vi "RT_VS50_Dynamics_DLR_v10_v11_PXI.vi"() -> ()   [LabVIEW 2017]
uses:
  <vilib>/Platform/TimedLoop/XDataNode/timing_clust.ctl
  <vilib>/Platform/TimedLoop/XDataNode/nitl_modes.ctl
  <vilib>/Platform/TimedLoop/XDataNode/wakeup.ctl
  <vilib>/Analysis/coordinate.llb/Euler Rotation Order.ctl
  <vilib>/Analysis/_algsub.llb/Vector Norm Type.ctl
  <vilib>/DAQmx/read.llb/DAQmx Read (Analog DBL 1Chan 1Samp).vi
  <vilib>/DAQmx/write.llb/DAQmx Write (Analog DBL 1Chan 1Samp).vi
  <vilib>/Analysis/baseanly.llb/Real A x B.vi
  <vilib>/Analysis/_algsub.llb/Real Vector Norm.vi
  <vilib>/Instr/_visa.llb/VISA Configure Serial Port (Instr).vi
  <vilib>/Utility/file.llb/Read Delimited Spreadsheet (DBL).vi
  <vilib>/DAQmx/create/channels.llb/DAQmx Create Channel (AO-Voltage-Basic).vi
  <vilib>/DAQmx/create/channels.llb/DAQmx Create Channel (AI-Voltage-Basic).vi
  <vilib>/DAQmx/miscellaneous.llb/DAQmx Fill In Error Info.vi
  <vilib>/Analysis/Matrix/Numeric/Conversions/Array To Matrix - RA2.vi
  <vilib>/Analysis/Matrix/Numeric/Conversions/Array To Matrix - RA.vi
  <vilib>/Analysis/Matrix/Numeric/Conversions/Matrix To Array - RM.vi
  <vilib>/Platform/TimedLoop/XDataNode/XDataNode.xnode
  <vilib>/Analysis/NI_AALPro.lvlib
  <vilib>/Platform/TimedLoop/XDataNode/XDNodeRunTimeDep.lvlib
  <vilib>/Utility/file.llb/Read From Spreadsheet File (DBL).vi
  <vilib>/Analysis/Matrix/NI_Matrix.lvlib
  <vilib>/Analysis/NI_AALBase.lvlib
  <vilib>/ptbypt/NI_PtbyPt.lvlib
panel:
  out "e (i+1)":cluster{dbl[], dbl[]}[](graph)
  out "all rows 2":dbl[][](array[numeric]) format="%0.3f"
  out "PID_array":dbl[][](array[numeric])
  in  "Guiamento":bool
  in  "Debug":bool
  in  "BR ACT - oscillation pitch":bool
  in  "BR ACT - oscillation yaw":bool
  in  "Amplitude [deg]":dbl=4.0 format="%#_13g"
  in  "Frequency [Hz]":dbl=1.0 format="%#_13g"
  out "BR ACT enable":bool
  in  "BR ACT - Enable Manual cmd":bool
  out "ACT Pitch [deg] mean":dbl format="%0.2f"
  out "ACT Yaw [deg] mean":dbl format="%0.2f"
  out "ACT Pitch [deg]":dbl
  out "ACT Yaw [deg]":dbl
  out "mean y":dbl format="%0.2f"
  out "mean x":dbl format="%0.2f"
  out "Incl angle Y [deg]":dbl
  out "Incl angle X [deg]":dbl
  out "Iteration Duration LOG":i64
  out "Iteration Duration CFG CFN":i64
  out "Iteration Duration NAV CFN":i64
  out "Iteration Duration sim [us]":i64
  out "LOG Enable":bool
  out "Table enable":bool
  out "DMARS Enable":bool
  out "TVA Enable":bool
  out "CFN-61G Enable":bool
  out "CRC?":bool
  out "string out":string
  in  "STIM300 Enable":bool
  out "CRC OK":bool
  out "IMU accel status":u8 format="%b"
  out "IMU incl status":u8 format="%b"
  out "Samples Counter":u8
  out "IMU gyro status":u8 format="%b"
  out "Inc X [g]":dbl
  out "Inc Y [g]":dbl
  out "Inc Z [g]":dbl
  out "Iteration Duration STIM":i64
  out "ACT Pitch read":dbl(slide) scale=0.0..5.0
  out "ACT Yaw read":dbl(slide) scale=0.0..5.0
  in  "Atuador Yaw [Deg]":dbl(knob) scale=-4.0..4.0
  in  "Atuador Pitch [Deg]":dbl(knob) scale=-4.0..4.0
  out "Iteration Duration ACT":i64
  in  "Simulation Parameters":T1={"Wind VelocityAzimuth [deg] "=0.0, "Wind Velocity Module [m/s]"=0.0, "Fe gain"=1.0, "Cnalpha gain"=1.0, "clp gain"=1.0, "cld gain"=1.0, "cmq gain"=1.0, "cnr gain"=1.0, "dl [º]"=0.0, "Nozzle misalignment yaw/pitch [º]"=[0.0, 0.0], "Nozzle eccentricity x/y [m]"=[], "Wind_Profile"=0} {"Wind_Profile" min=0 max=3 step=1; "Wind Velocity Module [m/s]" format="%#_13g"; "Wind VelocityAzimuth [deg]" format="%#_13g"}
  in  "Initialization Parameters":T2={"W_b ini [rad/s]"=[0.0, 0.0, 0.0], "W ini [rad/s]"=[0.0, 0.0, 0.0], "altitude_ini(m)"=50.0, "lon_ini [º]"=-44.36778, "latd_ini [º]"=-2.31599, "V_ini [m/s]"=[0.0, 0.0, 0.0], "Initial Euler Angles [deg]"=[0.0, 0.0, 0.0], "CFN-61G Enable"=FALSE, "Table enable"=FALSE, "DMARS Enable"=FALSE, "German TVA Enable"=FALSE, "Sim_Time [s]"=82.0, "Control Selection"=enum."Sim Control", "LOG Enable"=FALSE, "BR ACT enable"=FALSE}
  out "concatenated string 2":string
  out "PXI log path 2":path
  out "concatenated string":string
  out "appended path":path
  in  "UTC format":bool
  out "spreadsheet string":string
  out "Sim_Time [s]":dbl
  in  "Rotation":T3
  out "TVA_cmd [deg] 2":dbl[](array[numeric])
  out "Control Variables (extra variables)":dbl[](array[numeric])
  in  "Send":bool
  out "Table Ready":bool
  out "CIVITA as DMARS [º]":cluster{"phi":dbl, "theta":dbl, "psi":dbl}
  in  "Cluster":T4={"Offset Roll"=0.0, "Offset Pitch"=0.0, "Offset Heading"=0.0, "Azimuth"=0.0, "Latitude "=-23.213156, "Longitude"=-45.860622, "Height"=622.367, "LP_Vel_Z-North"=0.0, "LP_Vel_Y-East"=0.0, "LP_Vel_X-Up"=0.0}
  out "Table cmd [º] inner middle outer":dbl[](array[numeric])
  out "DMARS SIM pred[º]":cluster{"phi":dbl, "theta":dbl, "psi":dbl}
  out "Control Variables\n (extra variables)":dbl[](array[numeric])
  out "ACT 315 Angle \"Yaw\"":dbl(slide) scale=-3.0..3.0
  out "ACT 225 Angle \"Pitch\"":dbl(slide) scale=-3.0..3.0
  out "TVA string 2":string
  out "TVA bytes read 2":u32
  out "CRC Check over Byte #10 to byte #84":bool
  out "CRC Check over Byte #2 to Byte #7 TVA2BComp":bool
  out "Iteration Duration TBL":i64
  out "Roll Rate/angle":dbl[](array[numeric])
  out "CRC Check over Byte #2 to Byte #7":bool
  out "CRC Check over Byte #10 to byte #29":bool
  out "GC_Counter 2":u32
  out "string to write DMARS":string="*IDN?"
  out "TVA string":string
  out "TVA bytes read":u32
  out "TVA sync bytes":string
  out "Time (s)":dbl
  out "POS":cluster{dbl, dbl, dbl} {"?" format="%_6g"; "?" format="%#1_6g"}
  out "RATE":cluster{dbl, dbl, dbl} {"?" format="%1_6g"}
  out "ACCEL":cluster{dbl, dbl, dbl} {"?" format="%1_6g"}
  out "Period":i64
  out "string enviada para acutrol":string
  in  "Remote Host":string="192.168.53.1"
  out "XYZ - rate_CIVITA":sgl[](array[numeric])
  out "Opp_Mode_CIVITA":string
  in  "NavOn":bool
  in  "Init":bool
  out "Long_Lat_Alt_CIVITA":sgl[](array[numeric])
  out "Euler Angles_CIVITA":sgl[](array[numeric])
  out "all rows":dbl[][](array[numeric]) format="%0.3f"
  in  "Start_SIMULATION":bool
  out "Data 4":dbl[][](array[numeric])
  out "Data 3":dbl[][](array[numeric])
  out "Data 2":dbl[][](array[numeric])
  out "Current time [s]":dbl
  out "bad iteration":bool
  in  "stop RT":bool
  out "SIM_Running":bool
  # "atitudes após leveling"
  # "0.279817"
  # "0.119821"
  # "0.24729"
  # "-0.038932"
  # "-0.0385253"
  # "-0.038247"
  # "-0.0193609"
  # "-0.0178696"
  # "-0.0176574"
  # "Posicão inicial"
  # "Posicao after 10min"
  # "-45.8606"
  # "-48.1427"
  # "-23.2132"
  # "-23.2324"
  # "0.622374"
  # "-4.67869"
  # "INS Civitanavi Control"
  # "0xAA/ 0x55"
  # "830 steps"
  # "Reiniciar a vi sempre antes de uma nova simulação!!"
  # "Simulation"
  # "TVA COMMUNICATIONS (German HW)"
  # "Enable buttons"
  # "Motion simulation table Control and Log files"
  # "Housekeeping data"
  # "º"
  # "Command Data"
  # "º"
  # "Km"
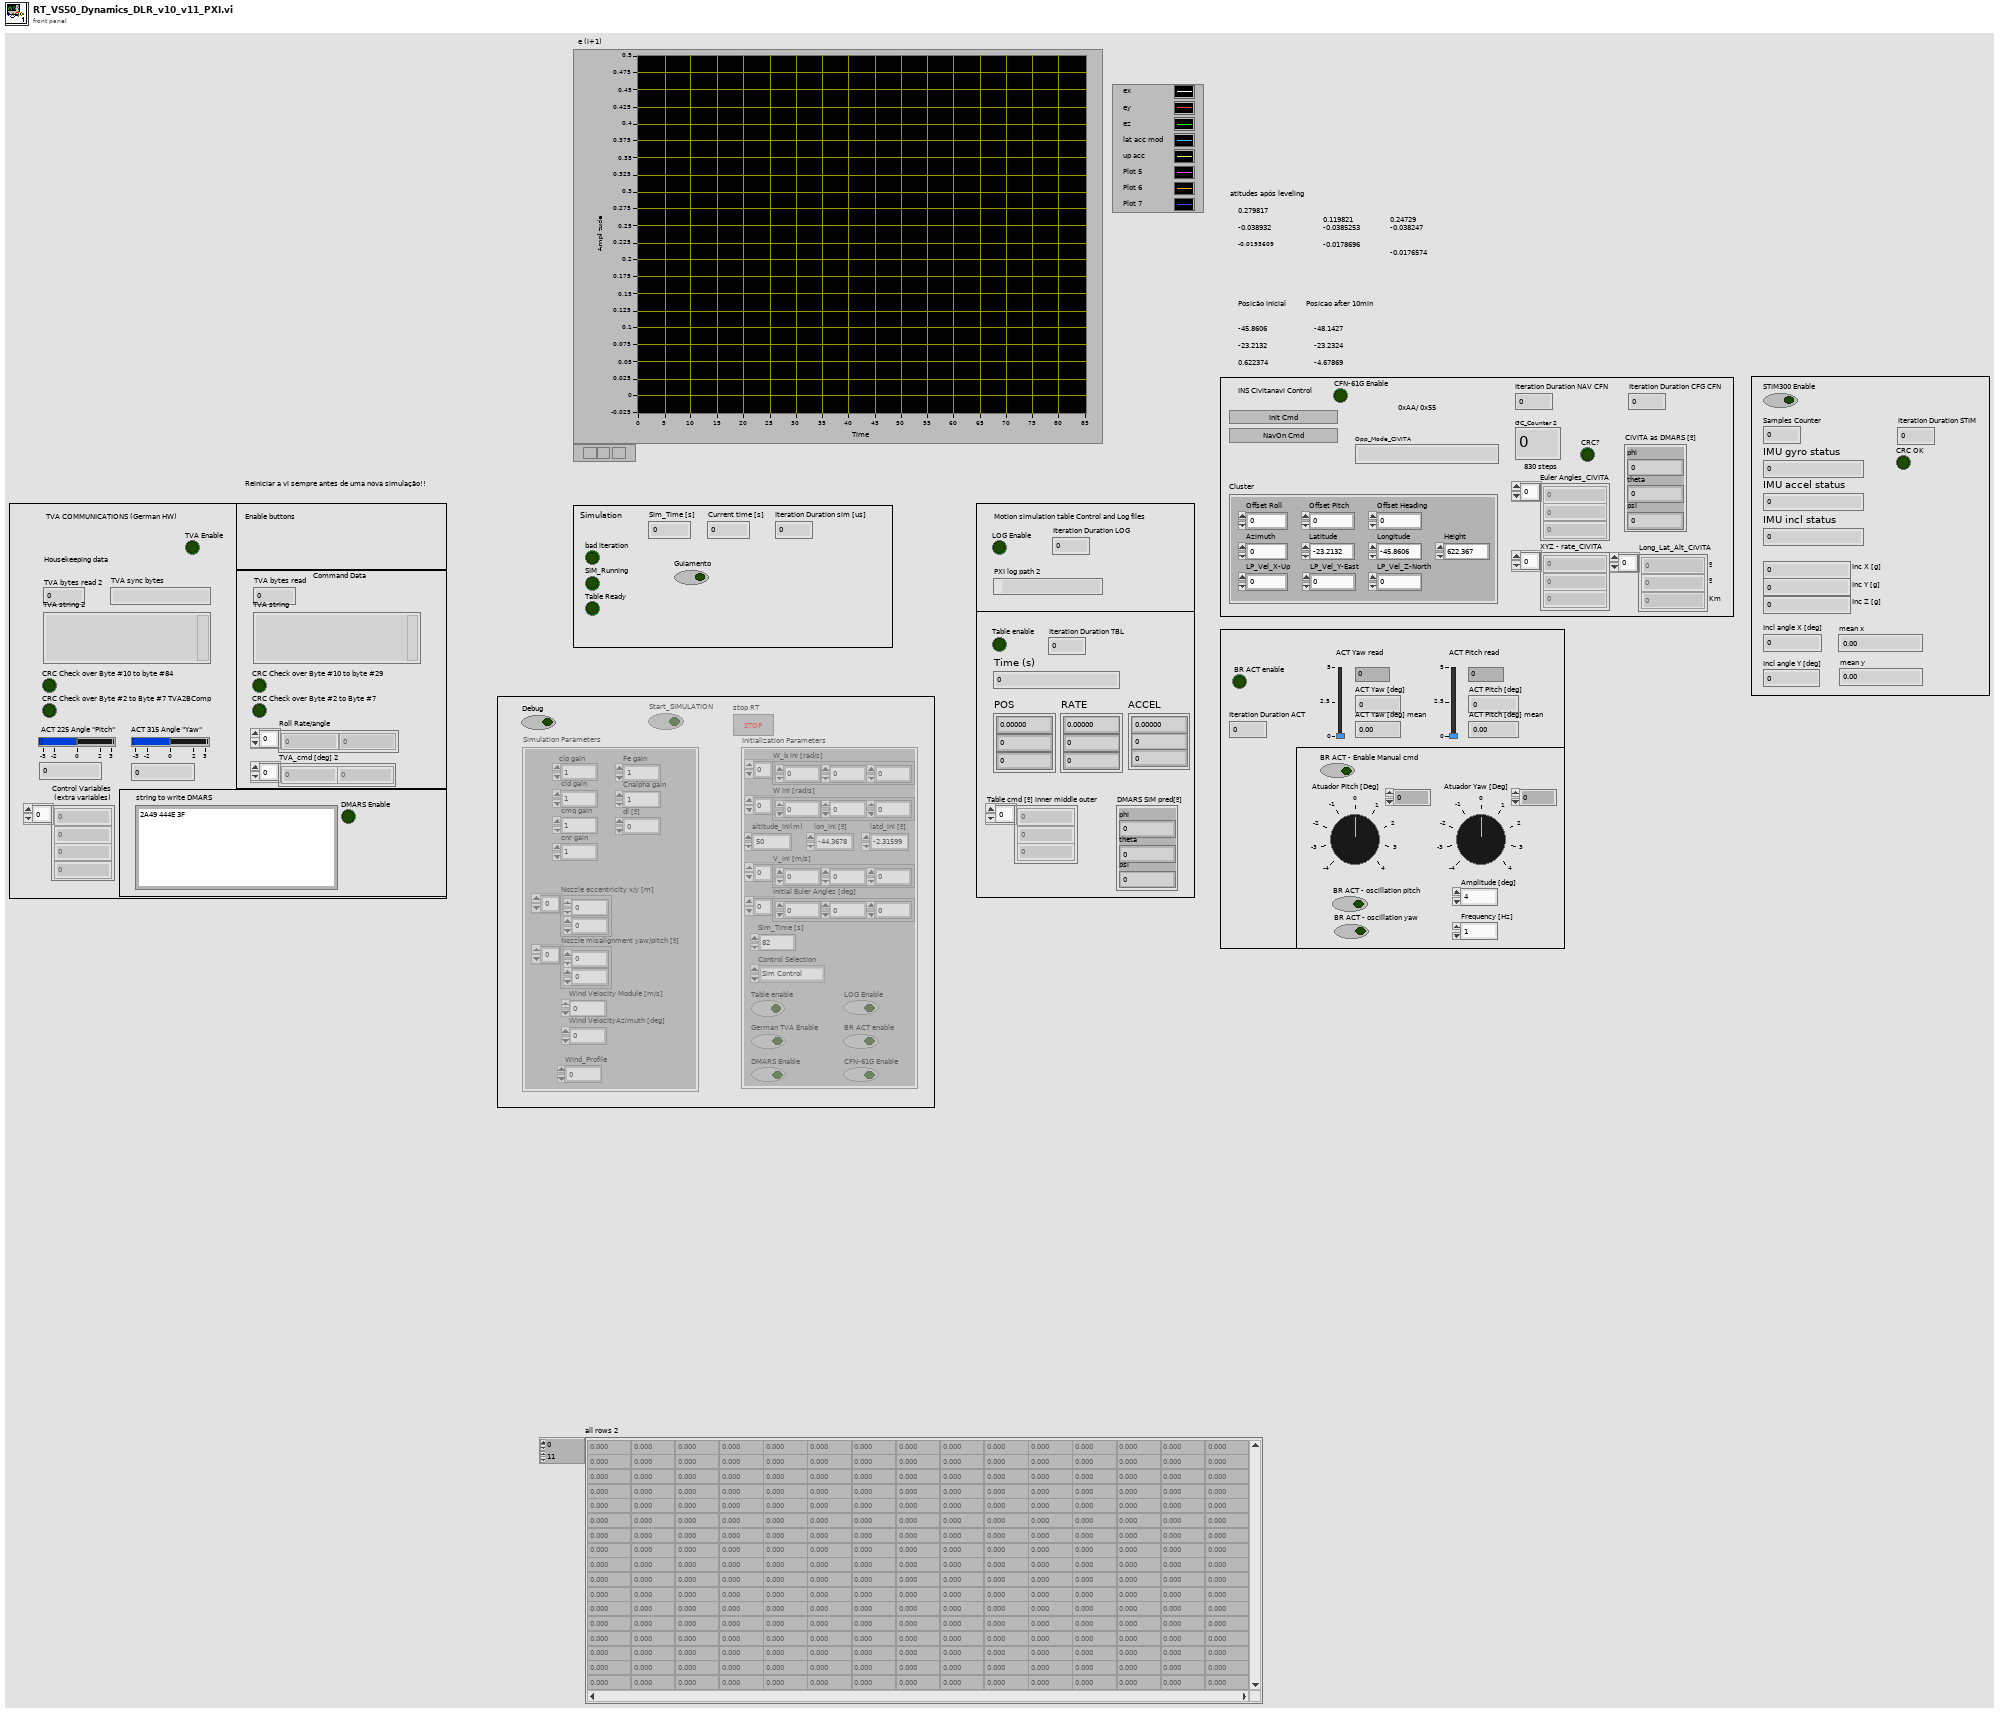
[diagram p1: front panel]
types:
  T1 = cluster{"Wind VelocityAzimuth [deg] ":dbl, "Wind Velocity Module [m/s]":dbl, "Fe gain":dbl, "Cnalpha gain":dbl, "clp gain":dbl, "cld gain":dbl, "cmq gain":dbl, "cnr gain":dbl, "dl [º]":dbl, "Nozzle misalignment yaw/pitch [º]":dbl[], "Nozzle eccentricity x/y [m]":dbl[], "Wind_Profile":i32}
  T2 = cluster{"W_b ini [rad/s]":dbl[], "W ini [rad/s]":dbl[], "altitude_ini(m)":dbl, "lon_ini [º]":dbl, "latd_ini [º]":dbl, "V_ini [m/s]":dbl[], "Initial Euler Angles [deg]":dbl[], "CFN-61G Enable":bool, "Table enable":bool, "DMARS Enable":bool, "German TVA Enable":bool, "Sim_Time [s]":dbl, "Control Selection":enum16{"Constant", "TVA E-BOX", "Sim Control"}, "LOG Enable":bool, "BR ACT enable":bool}
  T3 = cluster{"W(i) [rad/s]":dbl[], "W_b(i) [rad/s]":dbl[], "q(i)":dbl[], "Euler Angles {rad]":dbl[]}
  T4 = cluster{"Offset Roll":sgl, "Offset Pitch":sgl, "Offset Heading":sgl, "Azimuth":sgl, "Latitude ":sgl, "Longitude":sgl, "Height":sgl, "LP_Vel_Z-North":sgl, "LP_Vel_Y-East":sgl, "LP_Vel_X-Up":sgl}
  T5 = enum8{"Enabled", "Disabled", "Disabled and Grayed Out"}
  T6 = typedef "XDNodeRunTimeDep.lvlib/timing_clust.ctl" = cluster{"Expected End [f-1]":u64, "Actual End [f-1]":u64, "Finished Late? [f-1]":bool, "Expected End [i-1]":u64, "Actual End [i-1]":u64, "Finished Late? [i-1]":bool, "Expected Start [i]":u64, "Actual Start [i]":u64, "Expected Start [f]":u64, "Actual Start [f]":u64, "Source Name":string, "Structure Name":string, "Period":i64, "Deadline":i64, "Offset":i64, "Start":i64, "Priority":i32, "Timeout":i32, "Mode":T7, "Wakeup Reason":T8, "Error":errorcluster, "Source Type":string, "Secondary Source Type":string, "Global End Time":u64, "Global Start Time":u64, "Frame Duration":u64, "Iteration Duration":u64, "Assigned CPU":i32, "I/O Scan Engine Mode":u32}
  T7 = typedef "XDNodeRunTimeDep.lvlib/nitl_modes.ctl" = enum32{"No Change", "Process missed periods, maintain original phase", "Discard missed periods, maintain original phase", "Process missed periods, ignore original phase", "Discard missed periods, ignore original phase"}
  T8 = typedef "XDNodeRunTimeDep.lvlib/wakeup.ctl" = enum32{"Normal", "Aborted", "Asynchronous wakeup", "Timing source error", "Timed loop error", "Timeout"}
  T9 = cluster{"act_b [rad]":dbl[], "Oil Consumption [L]":dbl, "Act_b_TVA (315,225) [deg]":dbl[], "TVA cmd [rad]":dbl[], "BR ACT [rad]":dbl[]}
  T10 = cluster{"W(i+1) [rad/s]":dbl[], "W_b(i+1) [rad/s]":dbl[], "q(i+1)":dbl[], "Euler angles (i+1) XYZ [rad]":dbl[]}
  T11 = cluster{"position ECEF (i)":dbl[], "Lat_C [rad]":dbl, "latd(i+1) [rad]":dbl, "lon(i+1) [rad]":dbl, "height (i+1) [m]":dbl, "V(i+1) [m/s] NWU":dbl[]}
  T12 = cluster{"latd(i) [rad]":dbl, "lon(i) [rad]":dbl, "height(i)(m)":dbl, "V(i) [m/s] NWU":dbl[]}
  T13 = typedef "NI_AALPro.lvlib/Euler Rotation Order.ctl" = u16
  T14 = cluster{"dt [s]":dbl, "sim_running":bool, "t[s]":dbl, "i":i32}
  T15 = cluster{"Nzl_S [m^2]":dbl, "le [m]":dbl, "dl [rad]":dbl, "Dref[m]":dbl, "Sref [m^2]":dbl, "Nozzle misalignment yaw/pitch [º]":dbl[], "Nozzle eccentricity x/y [m]":dbl[]}
  T16 = typedef "NI_Matrix.lvlib/RealMatrix.ctl" = dbl[][]
  T17 = cluster{"output cluster":cluster{"AoA_pitch [rad]":dbl, "AoA_yaw [rad]":dbl, "Stream_direction [rad]":dbl[], "Speed_direction [rad]":dbl[]}, "M_alpha [rad/s^2], M_beta [rad/s^2]":cluster{"M_alpha [rad/s²]":dbl, "M_beta [rad/s²]":dbl}, "acc [m/s^2]":dbl[], "ang_acc":dbl[], "FE_b [N], FG [N], FA [N], Fco[N]":cluster{"FE_b [N]":dbl[], "FG [N]":dbl[], "FA [N]":dbl[], "Fco [N]":dbl[]}, "k_acc":cluster{"lat_acc_mod":dbl, "up_acc":dbl}}
  T18 = typedef "NI_AALPro.lvlib/Vector Norm Type.ctl" = u16
  T19 = enum16{"open", "replace", "create", "open or create", "replace or create", "replace or create with confirmation"}
  T20 = cluster{"Numeric":dbl, "upper limit":dbl, "upper limit":dbl}
  T21 = cluster{dbl, "upper limit":dbl, "upper limit":dbl}
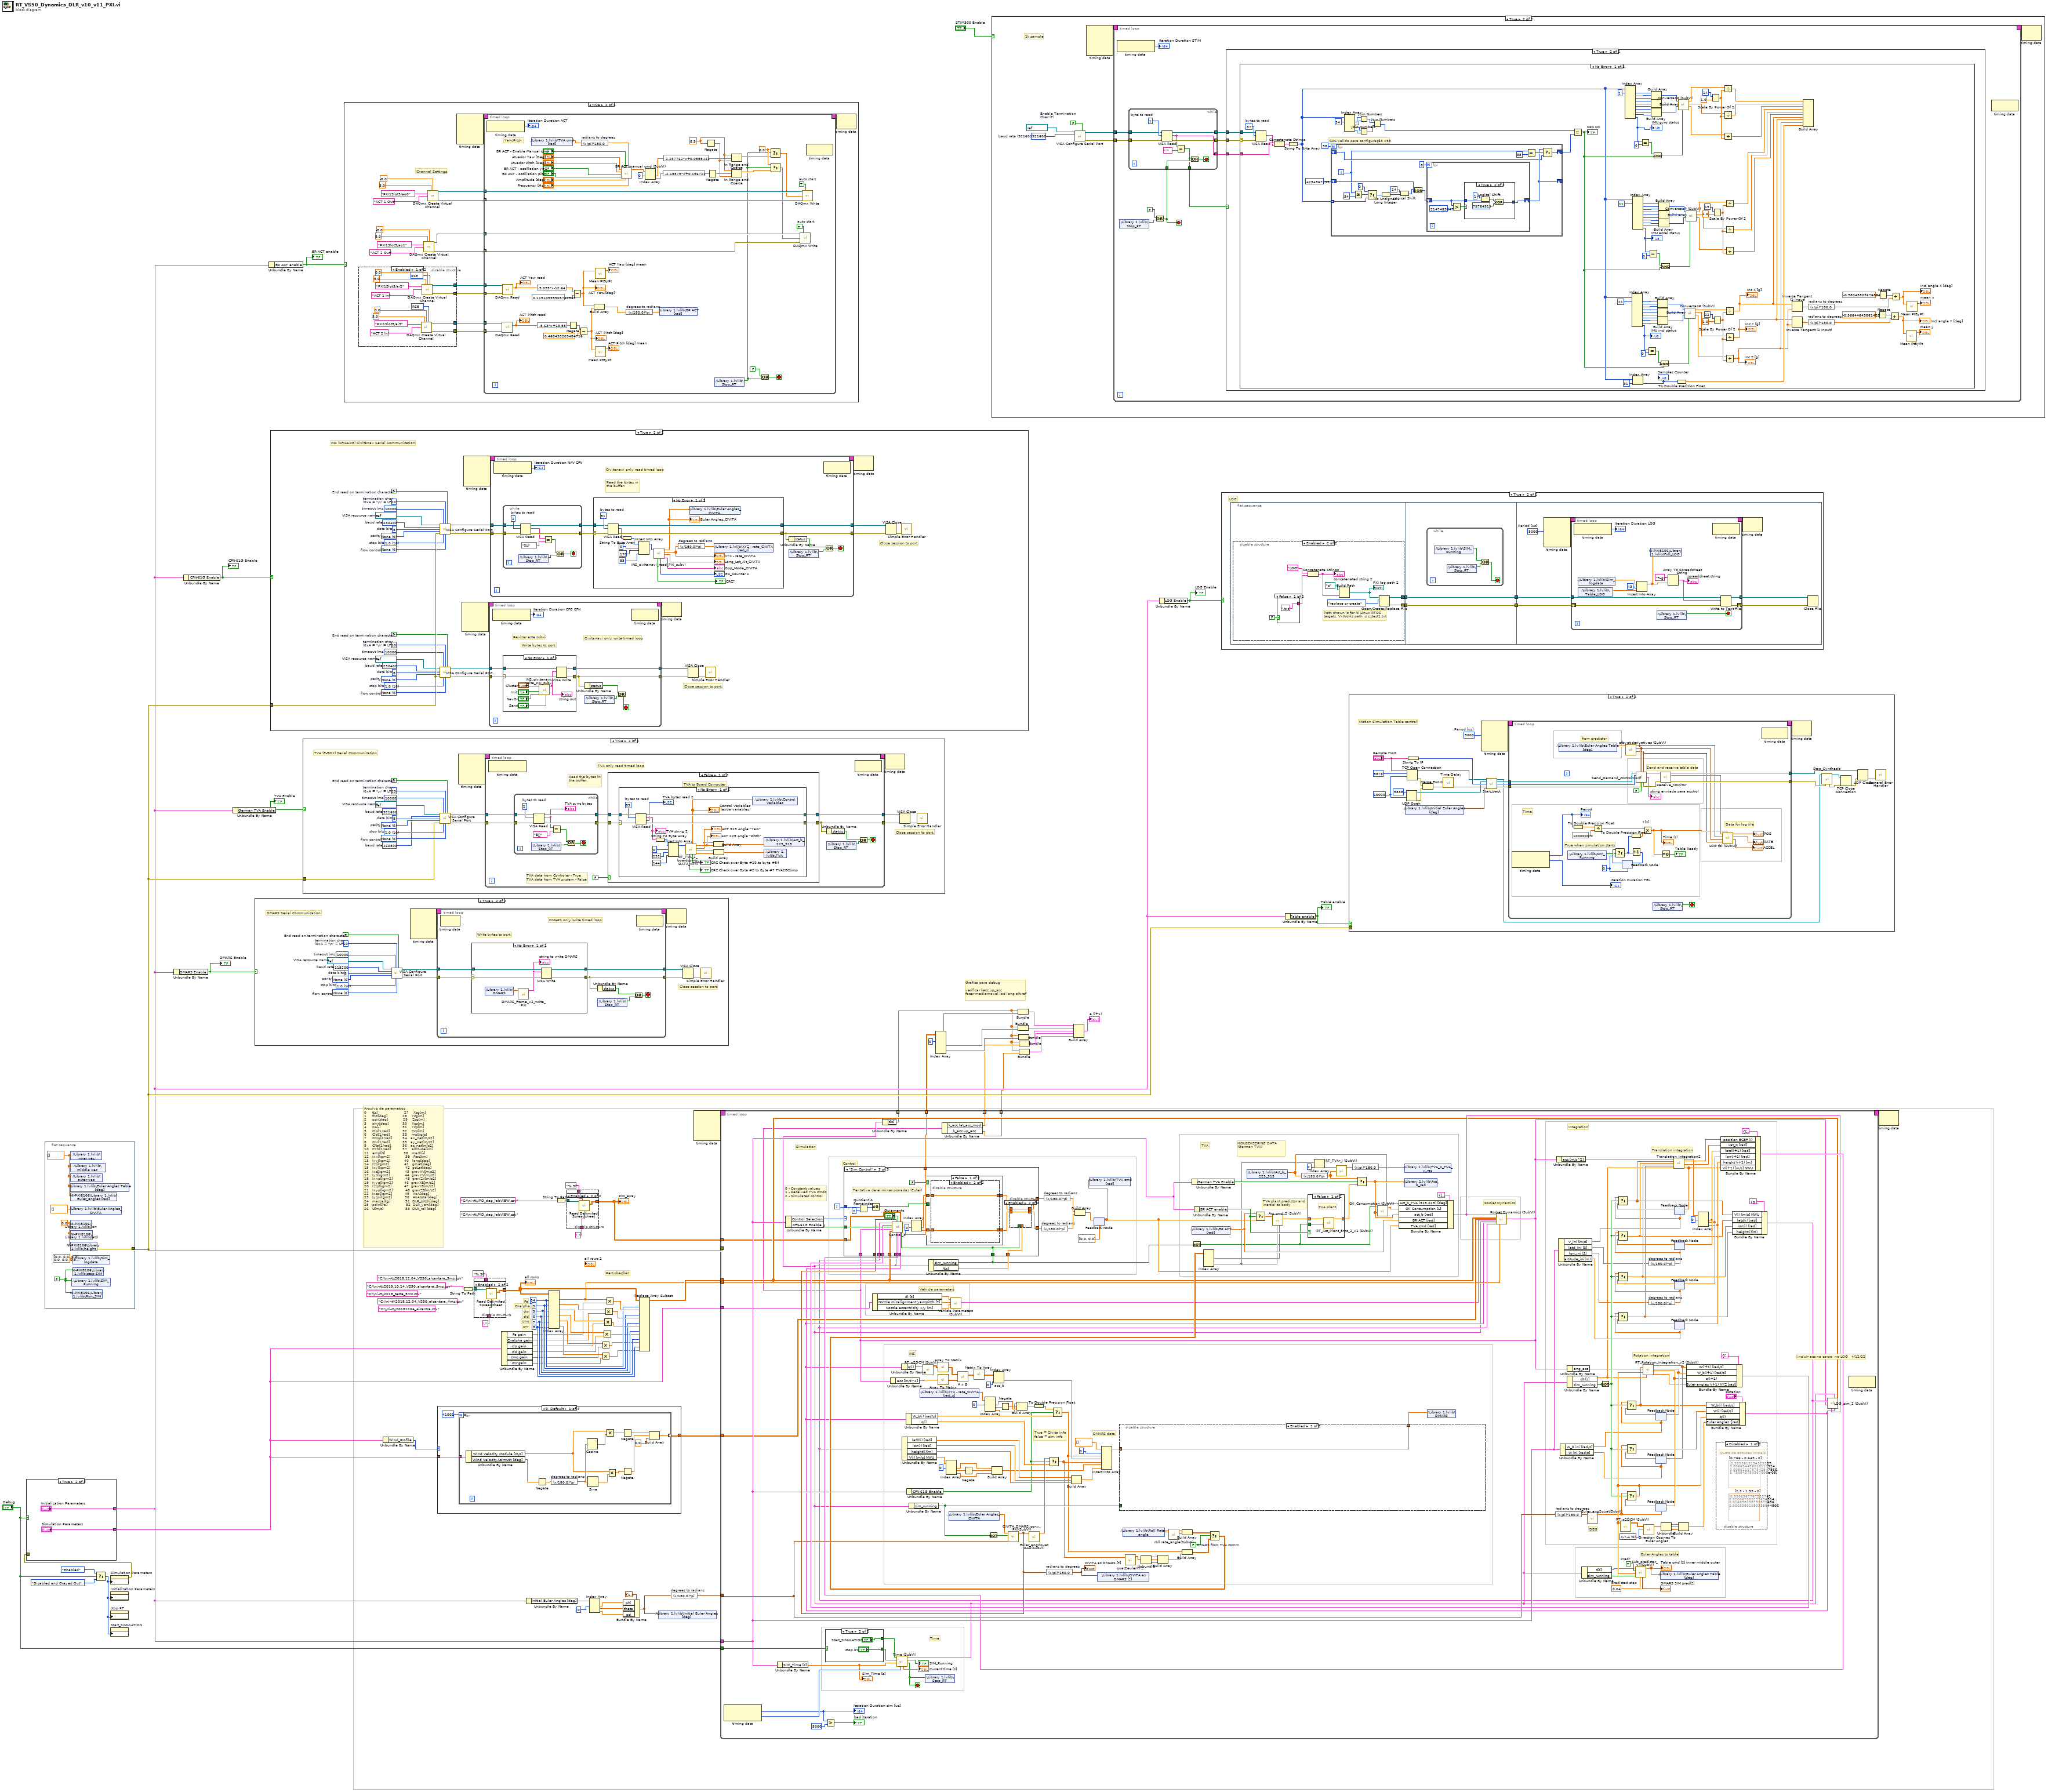
[diagram p0: block diagram]
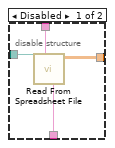
[diagram p2: hidden frame]
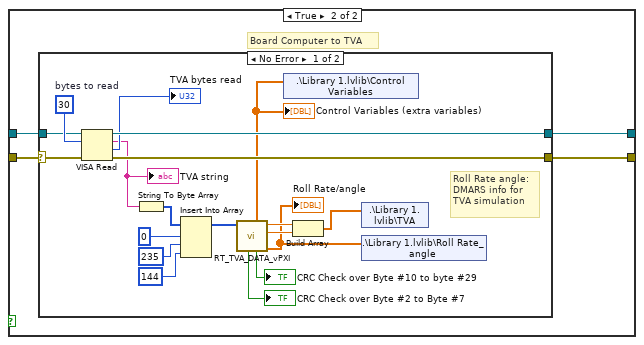
[diagram p9: hidden frame]
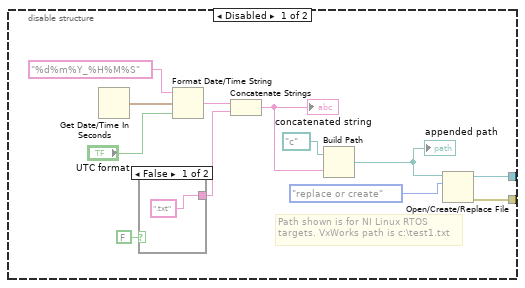
[diagram p12: hidden frame]
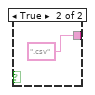
[diagram p13: hidden frame]
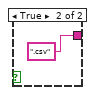
[diagram p14: hidden frame]
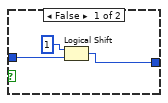
[diagram p18: hidden frame]
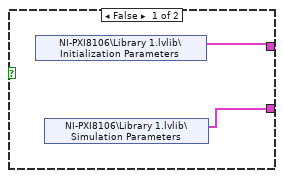
[diagram p20: hidden frame]
diagram:
  (unwired) "C:\\ni-rt\\PID_deg_labVIEW.csv"
  (unwired) "C:\\ni-rt\\2018_teste_5ms.csv"
  w57 = 8 ("index (col)")
  w58 = 7 ("index (col)")
  w59 = 6 ("index (col)")
  w63 = 5 ("index (col)")
  w66 = 9 ("index (col)")
  w70 = 54 ("disabled index (col)")
  (unwired) "C:\\ni-rt\\2018.12.04_VS50_alcantara_4ms.csv"
  (unwired) "C:\\ni-rt\\20181204_Alcantra.csv"
  (unwired) "C:\\ni-rt\\2018.12.04_VS50_alcantara_5ms.csv"
  # "Grafico para debug\n\nverificar kacc.up_acc\nfazer mediamovel lad long alt ref"
  # "Arquivo de parametros\n0     t[s]                       27    Xcg[m] \n1     thtr[deg]             28    Ycg[m]\n2     psir[deg]             29    Zcg[m]  \n3     phir[deg]            30    Xcp[m]       \n4     CA[-]                   31    Ycp[m]        \n5     Clp[1/rad]           32    Zcp[m]     \n6     Cld[1/rad]           33    mp[kg/s]        \n7     Cmq[1/rad]         34   ax_net[m/s2]         \n8     Cnr[1/rad]           35   ay_net[m/s2]      \n9     CNa[1/rad]          36   az_net[m/s2]      \n10   CYb[1/rad]          37    altitude[km]       \n11   emp[N]                38   mach[-]     \n12   Ixx[kgm2]             39   Rec[km]     \n13   Iyy[kgm2]            40   long[deg]     \n14   Izz[kgm2]             41   gcLat[deg]        \n15   Ixy[kgm2]             42  gdLat[deg]       \n16   Ixz[kgm2]             43  gravXV[m/s2]  \n17   Iyz[kgm2]             44  gravYV[m/s2]     \n18   Ixxp[kgm2]           45  gravZV[m/s2]         \n19   Iyyp[kgm2]          46  gravXB[m/s2]         \n20   Izzp[kgm2]           47  gravYB[m/s2]         \n21   Ixyp[kgm2]           48  gravZB[m/s2]           \n22   Ixzp[kgm2]           49   AoA[deg]             \n23   Iyzp[kgm2]           50   AoAtotal[deg]       \n24   massa[kg]             51  DLR_pitch[deg]    \n25   pdin[Pa]                52  DLR_yaw[deg]  \n26   U[m/s]                   53  DLR_roll[deg]"
  # "cnr"
  # "cmq"
  # "cld"
  # "clp"
  # "Cnalpha"
  # "Fe"
  # "Perturbações"
  n1 = flat-sequence {
    tunnel: [w80] -> w52
    frame #0 {
      w79 = dbl[] [] ("inner vec")
      w77 = FALSE ("SIM_Running")
      w82 = 0.0 ("lon")
      n2 = shared-variable ".\\Library 1.lvlib\\inner vec"(w79) -> ()  [unwired: 1 in, 1 out]
      n3 = shared-variable ".\\Library 1.lvlib\\middle vec"(w79) -> ()  [unwired: 1 in, 1 out]
      n4 = shared-variable ".\\Library 1.lvlib\\outer vec"(w79) -> ()  [unwired: 1 in, 1 out]
      n5 = shared-variable ".\\Library 1.lvlib\\Euler Angles Table [deg]"(w79) -> ()  [unwired: 1 in, 1 out]
      n6 = shared-variable "NI-PXI8106\\Library 1.lvlib\\Euler_angles [rad]"(w79) -> ()  [unwired: 1 in, 1 out]
      n7 = shared-variable ".\\Library 1.lvlib\\Euler Angles_CIVITA"(sgl[] [] ("Euler Angles_CIVITA")) -> ()  [unwired: 1 in, 1 out]
      n8 = shared-variable "NI-PXI8106\\Library 1.lvlib\\lon"(w82) -> ()  [unwired: 1 in, 1 out]
      n9 = shared-variable "NI-PXI8106\\Library 1.lvlib\\latd"(w82) -> ()  [unwired: 1 in, 1 out]
      n10 = shared-variable "NI-PXI8106\\Library 1.lvlib\\height"(w82) -> (error out=w80:errorcluster)  [unwired: 1 in]
      n11 = shared-variable ".\\Library 1.lvlib\\SIM_Running"(w77) -> ()  [unwired: 1 in, 1 out]
      n12 = shared-variable "NI-PXI8106\\Library 1.lvlib\\Run_SIM"(w77) -> ()  [unwired: 1 in, 1 out]
      n13 = shared-variable ".\\Library 1.lvlib\\Sim_logdata"(dbl[] [0.0, 0.0, 0.0, 0.0, 0.0, 0.0, 0.0, 0.0, 0.0, 0.0, 0.0, 0.0, 0.0, 0.0, 0.0, 0.0, 0.0, 0.0, 0.0, 0.0, 0.0, 0.0, 0.0, 0.0, 0.0, 0.0, 0.0, 0.0, 0.0, 0.0, 0.0, 0.0, 0.0] ("Sim_logdata")) -> ()  [unwired: 1 in, 1 out]
      n14 = shared-variable "NI-PXI8106\\Library 1.lvlib\\stop SIM"(w77) -> ()  [unwired: 1 in, 1 out]
    }
  }
  n15 = Select(t=T5."Enabled" ("Disabled"), s="Debug", f=T5."Disabled and Grayed Out" ("Disabled")) -> (s? t:f=w22:T5)
  n16 = property on="Simulation Parameters" class="Clust (strict)"("DisabledEnum"=w22) -> (error out=w23:errorcluster)  [unwired: 2 in, 1 out]
  n17 = case shown="True" "Debug" {
    tunnel: [w84 "Initialization Parameters"] -> w27
    tunnel: [w83 "Simulation Parameters"] -> w34
    tunnel: w23 -> [_ _]
    frame False {
      n18 = shared-variable "NI-PXI8106\\Library 1.lvlib\\Initialization Parameters"() -> (w84:T2)  [unwired: 1 in, 1 out]
      n19 = shared-variable "NI-PXI8106\\Library 1.lvlib\\Simulation Parameters"() -> (w83:T1)  [unwired: 1 in, 1 out]
    }
    frame True {
    }
  }
  n20 = property on="Initialization Parameters" class="Clust (strict)"("DisabledEnum"=w22) -> ()  [unwired: 2 in, 2 out]
  n21 = property on="stop RT" class="Bool"("DisabledEnum"=w22) -> ()  [unwired: 2 in, 2 out]
  n22 = property on="Start_SIMULATION" class="Bool (strict)"("DisabledEnum"=w22) -> ()  [unwired: 2 in, 2 out]
  n23 = Unbundle By Name(w27) -> ("DMARS Enable"=w45:bool)
  "DMARS Enable" <- w45
  n24 = Unbundle By Name(w27) -> ("CFN-61G Enable"=w31:bool)
  "CFN-61G Enable" <- w31
  n25 = Unbundle By Name(w27) -> ("German TVA Enable"=w44:bool)
  "TVA Enable" <- w44
  n26 = case shown="True" w45 {
    frame False {
    }
    frame True {
      w95 = u32 10000  # timeout (ms)
      w92 = u16 0 items=["None"=0, "XON/XOFF"=1, "RTS/CTS"=2, "DTR/DSR"=4]  # flow control
      w96 = u16 10 items=["1.0"=10, "1.5"=15, "2.0"=20]  # stop bits
      w97 = u16 0 items=["None", "Odd", "Even", "Mark", "Space"]  # parity
      w94 = FALSE  # End read on termination character?
      w93 = u8 10  # termination char (0xA = '\n' = LF)
      w91 = u16 8  # data bits
      w100 = u32 115200  # baud rate
      w99 = refnum<visa-resource-name> "COM3"  # VISA resource name
      # "DMARS Serial Communication"
      # "Close session to port."
      n27 = call-poly "VISA Configure Serial Port"("VISA resource name"=w99, "timeout (10sec)"=w95, "termination char\n(0xA = '\\n' = LF)"=w93, "Enable Termination\nChar (T)"=w94, "baud rate (9600)"=w100, "data bits (8)"=w91, "parity (0:none)"=w97, "stop bits (10: 1 bit)"=w96, "flow control (0:none)"=w92) -> ("VISA resource name out"=w88:refnum<visa-resource-name>, "error out"=w87:errorcluster)  [unwired: 1 in, 4 out]
      n28 = node-c288() -> (w102:T6)  [unwired: 4 in]
      n29 = timed-loop {
        tunnel: w87 -> [w107]
        tunnel: w88 -> [w108]
        tunnel: [w104] -> w90
        tunnel: [w103] -> w89
        timing: w102 -> [_]
        timing-out: [_] -> w101
        stop <- w106 stop-if-true
        # "Write bytes to port."
        # "DMARS only write timed loop"
        n30 = node-c288() -> ()  [unwired: 1 in, 1 out]
        n31 = case shown="No Error" w107 {
          selector: w107 -> [w112 w117]
          tunnel: [w115 w116] -> w104
          tunnel: [w114 w117] -> w103
          tunnel: w108 -> [w113 w116]
          frame No Error {
            n32 = shared-variable ".\\Library 1.lvlib\\DMARS"() -> (w111:dbl[])  [unwired: 1 in, 1 out]
            n33 = call "DMARS_Frame_v2_write_PXI.vi"("DMARS"=w111) -> ("string_Out"=w110:string)  [unwired: 9 in, 1 out]
            "string to write DMARS" <- w110
            n34 = VISA Write(VISA resource name=w113, write buffer=w110, error in (no error)=w112) -> (VISA resource name out=w115:refnum<visa-resource-name>, error out=w114:errorcluster)  [unwired: 1 out]
          }
          frame Error {
          }
        }
        n35 = Unbundle By Name(w103) -> ("status"=w109:bool)
        n36 = shared-variable ".\\Library 1.lvlib\\Stop_RT"() -> (w105:bool)  [unwired: 1 in, 1 out]
        n37 = Or(x=w109, y=w105) -> (x .or. y?=w106:bool)
        n38 = node-c288() -> ()  [unwired: 1 in, 1 out]
      }
      n39 = node-c288(w101) -> ()  [unwired: 1 out]
      n40 = VISA Close(VISA resource name=w90, error in (no error)=w89) -> (error out=w98:errorcluster)
      n41 = call <vilib>:"Simple Error Handler.vi"("error in (no error)"=w98) -> ()  [unwired: 1 in, 8 out]
    }
  }
  n42 = Unbundle By Name(w27) -> ("BR ACT enable"=w28:bool)
  "BR ACT enable" <- w28
  n43 = case shown="True" w31 {
    tunnel: w52 -> [_ w154]
    frame False {
    }
    frame True {
      w127 = u32 10000  # timeout (ms)
      w129 = u16 0 items=["None"=0, "XON/XOFF"=1, "RTS/CTS"=2, "DTR/DSR"=4]  # flow control
      w126 = u16 10 items=["1.0"=10, "1.5"=15, "2.0"=20]  # stop bits
      w125 = u16 0 items=["None", "Odd", "Even", "Mark", "Space"]  # parity
      w122 = FALSE  # End read on termination character?
      w128 = u8 10  # termination char (0xA = '\n' = LF)
      w130 = u16 8  # data bits
      w123 = u32 230400  # baud rate
      w124 = refnum<visa-resource-name> "COM4"  # VISA resource name
      w140 = u32 10000  # timeout (ms)
      w137 = u16 0 items=["None"=0, "XON/XOFF"=1, "RTS/CTS"=2, "DTR/DSR"=4]  # flow control
      w141 = u16 10 items=["1.0"=10, "1.5"=15, "2.0"=20]  # stop bits
      w142 = u16 0 items=["None", "Odd", "Even", "Mark", "Space"]  # parity
      w139 = FALSE  # End read on termination character?
      w138 = u8 10  # termination char (0xA = '\n' = LF)
      w136 = u16 8  # data bits
      w144 = u32 230400  # baud rate
      w143 = refnum<visa-resource-name> "COM3"  # VISA resource name
      # "Close session to port."
      # "Close session to port."
      # "INS (CFN-61G) Civitanav Serial Communication"
      n44 = call-poly "VISA Configure Serial Port"("VISA resource name"=w143, "timeout (10sec)"=w140, "termination char\n(0xA = '\\n' = LF)"=w138, "Enable Termination\nChar (T)"=w139, "baud rate (9600)"=w144, "data bits (8)"=w136, "parity (0:none)"=w142, "error in (no error)"=w154, "stop bits (10: 1 bit)"=w141, "flow control (0:none)"=w137) -> ("VISA resource name out"=w146:refnum<visa-resource-name>, "error out"=w145:errorcluster)  [unwired: 4 out]
      n45 = call-poly "VISA Configure Serial Port"("VISA resource name"=w124, "timeout (10sec)"=w127, "termination char\n(0xA = '\\n' = LF)"=w128, "Enable Termination\nChar (T)"=w122, "baud rate (9600)"=w123, "data bits (8)"=w130, "parity (0:none)"=w125, "error in (no error)"=w154, "stop bits (10: 1 bit)"=w126, "flow control (0:none)"=w129) -> ("VISA resource name out"=w134:refnum<visa-resource-name>, "error out"=w135:errorcluster)  [unwired: 4 out]
      n46 = node-c288() -> (w151:T6)  [unwired: 4 in]
      n47 = node-c288() -> (w153:T6)  [unwired: 4 in]
      n48 = timed-loop {
        timing: w151 -> [_]
        timing-out: [_] -> w150
        tunnel: w134 -> [w161]
        tunnel: [w158] -> w132
        tunnel: w135 -> [w162]
        tunnel: [w157] -> w133
        stop <- w156 stop-if-true
        # "Revisar este subvi"
        # "Write bytes to port."
        # "Civitanavi only write timed loop"
        n49 = node-c288() -> (→"Iteration Duration CFG CFN":i64)  [unwired: 1 in]
        n50 = case shown="No Error" w162 {
          selector: w162 -> [w168 w173]
          tunnel: [w171 w172] -> w158
          tunnel: [w170 w173] -> w157
          tunnel: w161 -> [w169 w172]
          frame No Error {
            n51 = call "INS_civitanavi_write_PXI_subvi.vi"("Send"="Send", "NavOn"="NavOn", "Init"="Init", "Cluster"="Cluster") -> ("string out"=w165:string)  [unwired: 7 in]
            "string out" <- w165
            n52 = VISA Write(VISA resource name=w169, write buffer=w165, error in (no error)=w168) -> (VISA resource name out=w171:refnum<visa-resource-name>, error out=w170:errorcluster)  [unwired: 1 out]
          }
          frame Error {
          }
        }
        n53 = Unbundle By Name(w157) -> ("status"=w160:bool)
        n54 = shared-variable ".\\Library 1.lvlib\\Stop_RT"() -> (w159:bool)  [unwired: 1 in, 1 out]
        n55 = Or(x=w160, y=w159) -> (x .or. y?=w156:bool)
        n56 = node-c288() -> ()  [unwired: 1 in, 1 out]
      }
      n57 = timed-loop {
        timing: w153 -> [_]
        timing-out: [_] -> w152
        tunnel: w146 -> [w186]
        tunnel: [w188] -> w148
        tunnel: w145 -> [w185]
        tunnel: [w187] -> w147
        stop <- w180 stop-if-true
        # "Read the bytes in the buffer."
        # "Civitanavi only read timed loop"
        n58 = node-c288() -> (→"Iteration Duration NAV CFN":i64)  [unwired: 1 in]
        n59 = while {
          tunnel: w186 -> [w217]
          tunnel: w185 -> [w216]
          tunnel: [w215] -> w182
          tunnel: [w214] -> w181
          stop <- w209 stop-if-true
          w218 = u32 2  # bytes to read
          n60 = shared-variable ".\\Library 1.lvlib\\Stop_RT"() -> (w211:bool)  [unwired: 1 in, 1 out]
          n61 = VISA Read(VISA resource name=w217, byte count=w218, error in (no error)=w216) -> (VISA resource name out=w215:refnum<visa-resource-name>, read buffer=w213:string, error out=w214:errorcluster)  [unwired: 1 out]
          n62 = Equal?(x=w213, y="ªU") -> (x = y?=w210:bool)
          n63 = Or(x=w210, y=w211) -> (x .or. y?=w209:bool)
        }
        n64 = case "Read bytes from port." shown="No Error" w181 {
          selector: w181 -> [w202 w207]
          tunnel: [w205 w207] -> w187
          tunnel: [w206 w208] -> w188
          tunnel: w182 -> [w203 w208]
          frame No Error {
            w204 = u32 91  # bytes to read
            n65 = VISA Read(VISA resource name=w203, byte count=w204, error in (no error)=w202) -> (VISA resource name out=w206:refnum<visa-resource-name>, read buffer=w201:string, error out=w205:errorcluster)  [unwired: 1 out]
            n66 = String To Byte Array(string=w201) -> (unsigned byte array=w197:u8[])
            n67 = Insert Into Array(array=w197, index=0, new element #1=u8 170 ("new element/subarray"), new element #2=u8 85 ("new element/subarray")) -> (w196:u8[])
            n68 = call "INS_civitanavi_read_PXI_subvi.vi"("U8_Input"=w196) -> ("Opp_Mode 2"=→"Opp_Mode_CIVITA":string, "Long_Lat_Alt"=→"Long_Lat_Alt_CIVITA":sgl[], "XYZ - rate"=w190:sgl[], "Euler Angles"=w200:sgl[], "GC_Counter 2"=→"GC_Counter 2":u32, "CRC?"=→"CRC?":bool)  [unwired: 4 in, 1 out]
            "Euler Angles_CIVITA" <- w200
            "XYZ - rate_CIVITA" <- w190
            n69 = expression code="(x/180.0)*pi" "degrees to radians"(w190) -> (w191:sgl[])
            n70 = shared-variable ".\\Library 1.lvlib\\Euler Angles_CIVITA"(w200) -> ()  [unwired: 1 in, 1 out]
            n71 = shared-variable ".\\Library 1.lvlib\\XYZ - rate_CIVITA [rad_s]"(w191) -> ()  [unwired: 1 in, 1 out]
          }
          frame Error {
            # "Error occurred \nreading Bytes at \nSerial Port"
          }
        }
        n72 = Unbundle By Name(w187) -> ("status"=w184:bool)
        n73 = shared-variable ".\\Library 1.lvlib\\Stop_RT"() -> (w183:bool)  [unwired: 1 in, 1 out]
        n74 = node-c288() -> ()  [unwired: 1 in, 1 out]
        n75 = Or(x=w184, y=w183) -> (x .or. y?=w180:bool)
      }
      n76 = node-c288(w150) -> ()  [unwired: 1 out]
      n77 = VISA Close(VISA resource name=w132, error in (no error)=w133) -> (error out=w131:errorcluster)
      n78 = call <vilib>:"Simple Error Handler.vi"("error in (no error)"=w131) -> ()  [unwired: 1 in, 8 out]
      n79 = node-c288(w152) -> ()  [unwired: 1 out]
      n80 = VISA Close(VISA resource name=w148, error in (no error)=w147) -> (error out=w149:errorcluster)
      n81 = call <vilib>:"Simple Error Handler.vi"("error in (no error)"=w149) -> ()  [unwired: 1 in, 8 out]
    }
  }
  n82 = case shown="True" w44 {
    tunnel: w52 -> [_ w224]
    frame False {
    }
    frame True {
      (unwired) u32 921600  # baud rate
      w230 = u32 10000  # timeout (ms)
      w233 = u16 0 items=["None"=0, "XON/XOFF"=1, "RTS/CTS"=2, "DTR/DSR"=4]  # flow control
      w229 = u16 10 items=["1.0"=10, "1.5"=15, "2.0"=20]  # stop bits
      w228 = u16 0 items=["None", "Odd", "Even", "Mark", "Space"]  # parity
      w231 = FALSE  # End read on termination character?
      w232 = u8 10  # termination char (0xA = '\n' = LF)
      w234 = u16 8  # data bits
      w225 = u32 460800  # baud rate
      w226 = refnum<visa-resource-name> "COM4"  # VISA resource name
      # "TVA (E-BOX) Serial Communication"
      # "Close session to port."
      n83 = call-poly "VISA Configure Serial Port"("VISA resource name"=w226, "timeout (10sec)"=w230, "termination char\n(0xA = '\\n' = LF)"=w232, "Enable Termination\nChar (T)"=w231, "baud rate (9600)"=w225, "data bits (8)"=w234, "parity (0:none)"=w228, "error in (no error)"=w224, "stop bits (10: 1 bit)"=w229, "flow control (0:none)"=w233) -> ("VISA resource name out"=w237:refnum<visa-resource-name>, "error out"=w238:errorcluster)  [unwired: 4 out]
      n84 = node-c288() -> (w240:T6)  [unwired: 4 in]
      n85 = timed-loop {
        tunnel: w238 -> [w245]
        tunnel: w237 -> [w246]
        tunnel: [w244] -> w235
        tunnel: [w243] -> w236
        timing: w240 -> [_]
        timing-out: [_] -> w239
        stop <- w242 stop-if-true
        # "Read the bytes in the buffer."
        # "TVA data from Controler - True\nTVA data from TVA system - False"
        # "TVA only read timed loop"
        n86 = node-c288() -> ()  [unwired: 1 in, 1 out]
        n87 = while {
          tunnel: w246 -> [w259]
          tunnel: w245 -> [w258]
          tunnel: [w257] -> w248
          tunnel: [w256] -> w247
          stop <- w251 stop-if-true
          w260 = u32 2  # bytes to read
          n88 = shared-variable ".\\Library 1.lvlib\\Stop_RT"() -> (w253:bool)  [unwired: 1 in, 1 out]
          n89 = VISA Read(VISA resource name=w259, byte count=w260, error in (no error)=w258) -> (VISA resource name out=w257:refnum<visa-resource-name>, read buffer=w255:string, error out=w256:errorcluster)  [unwired: 1 out]
          "TVA sync bytes" <- w255
          n90 = Equal?(x=w255, y="ë") -> (x = y?=w252:bool)
          n91 = Or(x=w252, y=w253) -> (x .or. y?=w251:bool)
        }
        n92 = case shown="False" FALSE ("TVA Protocol") {
          tunnel: w247 -> [w265 w291]
          tunnel: w248 -> [w266 w290]
          tunnel: [w263 w293] -> w243
          tunnel: [w264 w292] -> w244
          frame False {
            # "TVA to Board Computer"
            n93 = case "Read bytes from port." shown="No Error" w265 {
              selector: w265 -> [w283 w288]
              tunnel: [w286 w288] -> w263
              tunnel: [w287 w289] -> w264
              tunnel: w266 -> [w284 w289]
              frame No Error {
                w285 = u32 85  # bytes to read
                n94 = VISA Read(VISA resource name=w284, byte count=w285, error in (no error)=w283) -> (VISA resource name out=w287:refnum<visa-resource-name>, read buffer=w281:string, return count=→"TVA bytes read 2":u32, error out=w286:errorcluster)
                "TVA string 2" <- w281
                n95 = String To Byte Array(string=w281) -> (unsigned byte array=w280:u8[])
                n96 = Insert Into Array(array=w280, index=0, new element #1=u8 235 ("new element/subarray"), new element #2=u8 144 ("new element/subarray")) -> (w279:u8[])
                n97 = call "RT_TVA_2_boardcomp_DATA_vPXI.vi"("TVA data"=w279) -> ("TVA_Yaw [deg]"=w268:dbl, "TVA_Pitch [deg]"=w269:dbl, "Act 315 Angle \"Yaw\""=w271:dbl, "Act 225 Angle \"Pitch\""=w272:dbl, "CRC Check over Byte #10 to byte #84"=→"CRC Check over Byte #10 to byte #84":bool, "Control Variables (extra variables)"=w273:dbl[], "CRC Check over Byte #2 to Byte #7"=→"CRC Check over Byte #2 to Byte #7 TVA2BComp":bool)  [unwired: 4 in]
                "ACT 225 Angle \"Pitch\"" <- w272
                "ACT 315 Angle \"Yaw\"" <- w271
                "Control Variables\n (extra variables)" <- w273
                n98 = Build Array(w271, w272) -> (w270:dbl[])
                n99 = Build Array(w269, w268) -> (w267:dbl[])
                n100 = shared-variable ".\\Library 1.lvlib\\Control Variables"(w273) -> ()  [unwired: 1 in, 1 out]
                n101 = shared-variable ".\\Library 1.lvlib\\Act_b_225_315"(w270) -> ()  [unwired: 1 in, 1 out]
                n102 = shared-variable ".\\Library 1.lvlib\\TVA"(w267) -> ()  [unwired: 1 in, 1 out]
              }
              frame Error {
                # "Error occurred \nreading Bytes at \nSerial Port"
              }
            }
          }
          frame True {
            # "Board Computer to TVA"
            n103 = case "Read bytes from port." shown="No Error" w291 {
              selector: w291 -> [w308 w313]
              tunnel: [w311 w313] -> w293
              tunnel: [w312 w314] -> w292
              tunnel: w290 -> [w309 w314]
              frame No Error {
                w310 = u32 30  # bytes to read
                # "Roll Rate angle: \nDMARS info for \nTVA simulation"
                n104 = VISA Read(VISA resource name=w309, byte count=w310, error in (no error)=w308) -> (VISA resource name out=w312:refnum<visa-resource-name>, read buffer=w306:string, return count=→"TVA bytes read":u32, error out=w311:errorcluster)
                "TVA string" <- w306
                n105 = String To Byte Array(string=w306) -> (unsigned byte array=w305:u8[])
                n106 = Insert Into Array(array=w305, index=0, new element #1=u8 235 ("new element/subarray"), new element #2=u8 144 ("new element/subarray")) -> (w304:u8[])
                n107 = call "RT_TVA_DATA_vPXI.vi"("TVA data"=w304) -> ("Roll Rate/angle"=w294:dbl[], "Yaw Angle"=w299:dbl, "Pitch Angle"=w300:dbl, "CRC Check over Byte #10 to byte #29"=→"CRC Check over Byte #10 to byte #29":bool, "Control Variables (extra variables)"=w295:dbl[], "CRC Check over Byte #2 to Byte #7"=→"CRC Check over Byte #2 to Byte #7":bool)  [unwired: 5 in]
                "Roll Rate/angle" <- w294
                "Control Variables (extra variables)" <- w295
                n108 = shared-variable ".\\Library 1.lvlib\\Control Variables"(w295) -> ()  [unwired: 1 in, 1 out]
                n109 = Build Array(w300, w299) -> (w298:dbl[])
                n110 = shared-variable ".\\Library 1.lvlib\\TVA"(w298) -> ()  [unwired: 1 in, 1 out]
                n111 = shared-variable ".\\Library 1.lvlib\\Roll Rate_angle"(w294) -> ()  [unwired: 1 in, 1 out]
              }
              frame Error {
                # "Error occurred \nreading Bytes at \nSerial Port"
              }
            }
          }
        }
        n112 = Unbundle By Name(w243) -> ("status"=w249:bool)
        n113 = shared-variable ".\\Library 1.lvlib\\Stop_RT"() -> (w241:bool)  [unwired: 1 in, 1 out]
        n114 = node-c288() -> ()  [unwired: 1 in, 1 out]
        n115 = Or(x=w249, y=w241) -> (x .or. y?=w242:bool)
      }
      n116 = node-c288(w239) -> ()  [unwired: 1 out]
      n117 = VISA Close(VISA resource name=w235, error in (no error)=w236) -> (error out=w227:errorcluster)
      n118 = call <vilib>:"Simple Error Handler.vi"("error in (no error)"=w227) -> ()  [unwired: 1 in, 8 out]
    }
  }
  n119 = case shown="True" w28 {
    frame False {
    }
    frame True {
      # "Channel Settings"
      n120 = disable-structure shown="Enabled" {
        disable-tunnel: [w340 _] -> w320
        disable-tunnel: [w339 _] -> w319
        disable-tunnel: [w338 _] -> w318
        disable-tunnel: [w337 _] -> w317
        frame Enabled {
          w335 = 10083 items=["Default"=-1, "RSE"=10083, "NRSE"=10078, "Differential"=10106, "Pseudodifferential"=12529] ("input terminal configuration")
          w336 = 10083 items=["Default"=-1, "RSE"=10083, "NRSE"=10078, "Differential"=10106, "Pseudodifferential"=12529] ("input terminal configuration")
          n121 = call-poly <vilib>:"DAQmx Create Virtual Channel.vi"("maximum value"=5.0, "minimum value"=0.0, "input terminal configuration"=w335, "physical channels"=tag "PXI1Slot5/ai3", "name to assign"="ACT 2 In") -> ("task out"=w338:refnum<k21>, "error out"=w337:errorcluster)  [unwired: 9 in]
          n122 = call-poly <vilib>:"DAQmx Create Virtual Channel.vi"("maximum value"=5.0, "minimum value"=0.0, "input terminal configuration"=w336, "physical channels"=tag "PXI1Slot5/ai2", "name to assign"="ACT 1 In") -> ("task out"=w340:refnum<k21>, "error out"=w339:errorcluster)  [unwired: 9 in]
        }
        frame Disabled {
        }
      }
      n123 = call-poly <vilib>:"DAQmx Create Virtual Channel.vi"("maximum value"=8.0, "minimum value"=-8.0, "physical channels"=tag "PXI1Slot5/ao1", "name to assign"="ACT 2 Out") -> ("task out"=w322:refnum<k21>, "error out"=w321:errorcluster)  [unwired: 10 in]
      n124 = call-poly <vilib>:"DAQmx Create Virtual Channel.vi"("maximum value"=8.0, "minimum value"=-8.0, "physical channels"=tag "PXI1Slot5/ao0", "name to assign"="ACT 1 Out") -> ("task out"=w328:refnum<k21>, "error out"=w327:errorcluster)  [unwired: 10 in]
      n125 = node-c288() -> (w334:T6)  [unwired: 4 in]
      n126 = timed-loop {
        timing: w334 -> [_]
        timing-out: [_] -> w333
        tunnel: w328 -> [w395]
        tunnel: w327 -> [w394]
        tunnel: w322 -> [w392]
        tunnel: w321 -> [w391]
        tunnel: w320 -> [w389]
        tunnel: w319 -> [w388]
        tunnel: w318 -> [w387]
        tunnel: w317 -> [w386]
        stop <- w398 stop-if-true
        w368 = 0.0 ("t")
        w370 = 6.5 ("upper limit")
        w393 = TRUE  # auto start
        w396 = TRUE  # auto start
        # "Yaw/Pitch"
        n127 = node-c288() -> (→"Iteration Duration ACT":i64)  [unwired: 1 in]
        n128 = call-poly <vilib>:"DAQmx Read.vi"("task/channels in"=w387, "error in"=w386) -> ("data"=w384:dbl)  [unwired: 11 in, 2 out]
        "ACT Pitch read" <- w384
        n129 = call-poly <vilib>:"DAQmx Read.vi"("task/channels in"=w389, "error in"=w388) -> ("data"=w385:dbl)  [unwired: 11 in, 2 out]
        "ACT Yaw read" <- w385
        n130 = shared-variable ".\\Library 1.lvlib\\TVA cmd [rad]"() -> (w380:dbl[])  [unwired: 1 in, 1 out]
        n131 = expression code="5.035*x-12.64"(w385) -> (w363:dbl)
        n132 = expression code="-5.63*x+13.55"(w384) -> (w383:dbl)
        n133 = Negate(x=w383) -> (-x=w360:dbl)
        n134 = Subtract(x=w363, y=0.11510599905742565 ("ACT Yaw [deg] mean 2")) -> (x-y=w361:dbl)
        "ACT Yaw [deg]" <- w361
        n135 = Subtract(x=w360, y=0.468493209484716 ("ACT Pitch [deg] mean 2")) -> (x-y=w350:dbl)
        "ACT Pitch [deg]" <- w350
        n136 = expression code="(x/pi)*180.0" "radians to degrees"(w380) -> (w358:dbl[])
        n137 = Build Array(w361, w350) -> (w374:dbl[])
        n138 = call <vilib>:"Mean PtByPt.vi"("x"=w350) -> ("mean"=→"ACT Pitch [deg] mean":dbl)  [unwired: 3 in, 1 out]
        n139 = call <vilib>:"Mean PtByPt.vi"("x"=w361) -> ("mean"=→"ACT Yaw [deg] mean":dbl)  [unwired: 3 in, 1 out]
        n140 = call "BR ACT manual cmd (SubVI).vi"("freq"="Frequency [Hz]", "Array of Double in"=w358, "amp"="Amplitude [deg]", "BR ACT - Manual cmd"="BR ACT - Enable Manual cmd", "BR ACT - Manual cmd osc p"="BR ACT - oscillation pitch", "BR ACT - Manual cmd osc y"="BR ACT - oscillation yaw", "Atuador Pitch [Deg]"="Atuador Pitch [Deg]", "Atuador Yaw [Deg]"="Atuador Yaw [Deg]") -> ("Array of Double out"=w375:dbl[])  [unwired: 3 in]
        n141 = expression code="(x/180.0)*pi" "degrees to radians"(w374) -> (w373:dbl[])
        n142 = Index Array(array=w375, index #1=0 ("index")) -> (element #1=w378:dbl, element #2=w377:dbl)  [unwired: 1 in]
        n143 = shared-variable ".\\Library 1.lvlib\\BR ACT [rad]"(w373) -> ()  [unwired: 1 in, 1 out]
        n144 = expression code="-2.18579*x+0.196721"(w377) -> (w376:dbl)
        n145 = expression code="2.237762*x+0.0559441"(w378) -> (w372:dbl)
        n146 = Negate(x=w370) -> (-x=w369:dbl)
        n147 = Negate(x=w376) -> (-x=w371:dbl)
        n148 = shared-variable ".\\Library 1.lvlib\\Stop_RT"() -> (w349:bool)  [unwired: 1 in, 1 out]
        n149 = In Range and Coerce(upper limit=w370, x=w372, lower limit=w369) -> (coerced(x)=w367:dbl)  [unwired: 1 out]
        n150 = In Range and Coerce(upper limit=w370, x=w371, lower limit=w369) -> (coerced(x)=w365:dbl)  [unwired: 1 out]
        n151 = Or(x=FALSE, y=w349) -> (x .or. y?=w398:bool)
        n152 = Select(t=w368, s=w349, f=w367) -> (s? t:f=w366:dbl)
        n153 = Select(t=w368, s=w349, f=w365) -> (s? t:f=w364:dbl)
        n154 = call-poly <vilib>:"DAQmx Write.vi"("task/channels in"=w392, "auto start"=w393, "data"=w364, "error in"=w391) -> ()  [unwired: 9 in, 3 out]
        n155 = call-poly <vilib>:"DAQmx Write.vi"("task/channels in"=w395, "auto start"=w396, "data"=w366, "error in"=w394) -> ()  [unwired: 9 in, 3 out]
        n156 = node-c288() -> ()  [unwired: 1 in, 1 out]
      }
      n157 = node-c288(w333) -> ()  [unwired: 1 out]
    }
  }
  n158 = Unbundle By Name(w34) -> ("Wind_Profile"=w43:i32)
  n159 = case shown="0, Default" w43 {
    tunnel: [w405 w420 w433 w446] -> w72
    tunnel: w34 -> [w404 _ _ _]
    frame 0, Default {
      n160 = for {
        N: 41001 -> [_]
        tunnel: [w419] -> w405 mode=indexing
        tunnel: w404 -> [w409]
        n161 = Unbundle By Name(w409) -> ("Wind Velocity Module [m/s]"=w408:dbl, "Wind VelocityAzimuth [deg]"=w407:dbl)
        n162 = Negate(x=w407) -> (-x=w410:dbl)
        n163 = expression code="(x/180.0)*pi" "degrees to radians"(w410) -> (w411:dbl)
        n164 = Cosine(x=w411) -> (cos(x)=w417:dbl)
        n165 = Sine(x=w411) -> (sin(x)=w414:dbl)
        n166 = Multiply(x=w408, y=w417) -> (x*y=w416:dbl)
        n167 = Multiply(x=w408, y=w414) -> (x*y=w413:dbl)
        n168 = Negate(x=w416) -> (-x=w415:dbl)
        n169 = Negate(x=w413) -> (-x=w412:dbl)
        n170 = Build Array(w415, w412, 0.0 ("element")) -> (w419:dbl[])
      }
    }
    frame 1 {
      # "Carrega arquivo"
      n171 = String To Path(string="C:\\ni-rt\\vento_1_200hz.csv") -> (path=w423:path)
      n172 = disable-structure shown="Enabled" {
        disable-tunnel: "%.9f" ("format (%.3f)") -> [w428 w432]
        disable-tunnel: w423 -> [w427 w431]
        disable-tunnel: "," ("delimiter (\\t)") -> [w426 w429]
        disable-tunnel: [w425 w430] -> w420
        frame Disabled {
          n173 = call-poly <vilib>:"Read From Spreadsheet File.vi"("delimiter (\\t)"=w426, "format (%.3f)"=w428, "file path (dialog if empty)"=w427) -> ("all rows"=w425:dbl[][])  [unwired: 4 in, 4 out]
        }
        frame Enabled {
          n174 = call-poly <vilib>:"Read Delimited Spreadsheet.vi"("file path (dialog if empty)"=w431, "format (%.3f)"=w432, "delimiter (\\t)"=w429) -> ("all rows"=w430:dbl[][])  [unwired: 7 in, 5 out]
        }
      }
      "Data 2" <- w420
    }
    frame 2 {
      # "Carrega arquivo"
      n175 = String To Path(string="C:\\ni-rt\\vento_2_200hz.csv") -> (path=w436:path)
      n176 = disable-structure shown="Enabled" {
        disable-tunnel: "%.9f" ("format (%.3f)") -> [w441 w445]
        disable-tunnel: w436 -> [w440 w444]
        disable-tunnel: "," ("delimiter (\\t)") -> [w439 w442]
        disable-tunnel: [w438 w443] -> w433
        frame Disabled {
          n177 = call-poly <vilib>:"Read From Spreadsheet File.vi"("delimiter (\\t)"=w439, "format (%.3f)"=w441, "file path (dialog if empty)"=w440) -> ("all rows"=w438:dbl[][])  [unwired: 4 in, 4 out]
        }
        frame Enabled {
          n178 = call-poly <vilib>:"Read Delimited Spreadsheet.vi"("file path (dialog if empty)"=w444, "format (%.3f)"=w445, "delimiter (\\t)"=w442) -> ("all rows"=w443:dbl[][])  [unwired: 7 in, 5 out]
        }
      }
      "Data 3" <- w433
    }
    frame 3 {
      # "Carrega arquivo"
      n179 = String To Path(string="C:\\ni-rt\\vento_4_200hz.csv") -> (path=w448:path)
      n180 = disable-structure shown="Enabled" {
        disable-tunnel: "%.9f" ("format (%.3f)") -> [w454 w458]
        disable-tunnel: w448 -> [w453 w457]
        disable-tunnel: "," ("delimiter (\\t)") -> [w452 w455]
        disable-tunnel: [w451 w456] -> w446
        frame Disabled {
          n181 = call-poly <vilib>:"Read From Spreadsheet File.vi"("delimiter (\\t)"=w452, "format (%.3f)"=w454, "file path (dialog if empty)"=w453) -> ("all rows"=w451:dbl[][])  [unwired: 4 in, 4 out]
        }
        frame Enabled {
          n182 = call-poly <vilib>:"Read Delimited Spreadsheet.vi"("file path (dialog if empty)"=w457, "format (%.3f)"=w458, "delimiter (\\t)"=w455) -> ("all rows"=w456:dbl[][])  [unwired: 7 in, 5 out]
        }
      }
      "Data 4" <- w446
    }
  }
  n183 = String To Path(string="C:\\ni-rt\\2019.10.14_VS50_alcantara_5ms.csv") -> (path=w53:path)
  n184 = disable-structure shown="Enabled" {
    disable-tunnel: "," ("delimiter (\\t)") -> [w462 w464]
    disable-tunnel: "%.9f" ("format (%.3f)") -> [w461 w465]
    disable-tunnel: [w460 w463] -> w69
    disable-tunnel: w53 -> [w459 w466]
    frame Disabled {
      n185 = call-poly <vilib>:"Read From Spreadsheet File.vi"("delimiter (\\t)"=w462, "format (%.3f)"=w461, "file path (dialog if empty)"=w459) -> ("all rows"=w460:dbl[][])  [unwired: 4 in, 4 out]
    }
    frame Enabled {
      n186 = call-poly <vilib>:"Read Delimited Spreadsheet.vi"("file path (dialog if empty)"=w466, "format (%.3f)"=w465, "delimiter (\\t)"=w464) -> ("all rows"=w463:dbl[][])  [unwired: 7 in, 5 out]
    }
  }
  "all rows" <- w69
  n187 = Unbundle By Name(w34) -> ("Fe gain"=w42:dbl, "Cnalpha gain"=w41:dbl, "clp gain"=w40:dbl, "cld gain"=w39:dbl, "cmq gain"=w38:dbl, "cnr gain"=w37:dbl)
  n188 = Unbundle By Name(w27) -> ("Initial Euler Angles [deg]"=w50:dbl[])
  n189 = Index Array(array=w69, index (col) #1=w70, index (col) #2=w66, index (col) #3=w63, index (col) #4=w59, index (col) #5=w58, index (col) #6=w57) -> (element #1=w21:dbl[], element #2=w68:dbl[], element #3=w65:dbl[], element #4=w61:dbl[], element #5=w60:dbl[], element #6=w62:dbl[])  [unwired: 6 in]
  n190 = String To Path(string="C:\\ni-rt\\IPD_deg_labVIEW.csv") -> (path=w20:path)
  n191 = disable-structure shown="Enabled" {
    disable-tunnel: "," ("delimiter (\\t)") -> [w470 w472]
    disable-tunnel: "%.9f" ("format (%.3f)") -> [w469 w473]
    disable-tunnel: [w468 w471] -> w17
    disable-tunnel: w20 -> [w467 w474]
    frame Disabled {
      n192 = call-poly <vilib>:"Read From Spreadsheet File.vi"("delimiter (\\t)"=w470, "format (%.3f)"=w469, "file path (dialog if empty)"=w467) -> ("all rows"=w468:dbl[][])  [unwired: 4 in, 4 out]
    }
    frame Enabled {
      n193 = call-poly <vilib>:"Read Delimited Spreadsheet.vi"("file path (dialog if empty)"=w474, "format (%.3f)"=w473, "delimiter (\\t)"=w472) -> ("all rows"=w471:dbl[][])  [unwired: 7 in, 5 out]
    }
  }
  "PID_array" <- w17
  n194 = Index Array(array=w50, index #1=0 ("index")) -> (element #1=w48:dbl, element #2=w46:dbl, element #3=w47:dbl)  [unwired: 2 in]
  n195 = Multiply(x=w60, y=w38) -> (x*y=w55:dbl[])
  n196 = Multiply(x=w62, y=w37) -> (x*y=w54:dbl[])
  n197 = Multiply(x=w61, y=w39) -> (x*y=w56:dbl[])
  n198 = Multiply(x=w65, y=w40) -> (x*y=w64:dbl[])
  n199 = Multiply(x=w68, y=w41) -> (x*y=w67:dbl[])
  n200 = Multiply(x=w21, y=w42) -> (x*y=w71:dbl[])
  n201 = Bundle By Name(cluster=cluster{"phi":dbl, "theta":dbl, "psi":dbl} {"phi"=1.532, "theta"=1.286, "psi"=0.0} ("Initial Euler Angles [deg]"), "phi"=w48, "theta"=w46, "psi"=w47) -> (w36:cluster{"phi":dbl, "theta":dbl, "psi":dbl})
  n202 = Replace Array Subset(array=w69, new element #1=w71, index (col) #1=w70, new element #2=w67, index (col) #2=w66, new element #3=w64, index (col) #3=w63, new element #4=w56, index (col) #4=w59, new element #5=w55, index (col) #5=w58, new element #6=w54, index (col) #6=w57) -> (w30:dbl[][])  [unwired: 6 in]
  n203 = shared-variable ".\\Library 1.lvlib\\Initial Euler Angles [deg]"(w36) -> ()  [unwired: 1 in, 1 out]
  n204 = expression code="(x/180.0)*pi" "degrees to radians"(w36) -> (w35:cluster{"phi":dbl, "theta":dbl, "psi":dbl})
  n205 = node-c288() -> (w76:T6)  [unwired: 4 in]
  n206 = timed-loop {
    timing: w76 -> [_]
    timing-out: [_] -> w75
    tunnel: w30 -> [w487]
    tunnel: w72 -> [w486]
    tunnel: w52 -> [_]
    tunnel: w35 -> [w528]
    tunnel: w27 -> [w490]
    tunnel: w34 -> [w539]
    tunnel: "Debug" -> [w519]
    tunnel: w21 -> [w482]
    tunnel: w17 -> [w481]
    tunnel: [w480] -> w14 mode=indexing
    tunnel: [w478] -> w1 mode=indexing
    tunnel: [w476] -> w5 mode=indexing
    tunnel: [w475] -> w4 mode=indexing
    i -> [w584]
    stop <- w524 stop-if-true
    w623 = 0.04  # predicted step
    w547 = FALSE  # DMARS from TVA comm
    w589 = TRUE  # Pred?
    w644 = T13 0 items=["X-Y-Z", "X-Z-Y", "Y-X-Z", "Y-Z-X", "Z-X-Y", "Z-Y-X", "X-Y-X", "X-Z-X", "Y-X-Y", "Y-Z-Y", "Z-X-Z", "Z-Y-Z"] ("rotation order")
    # "incluir acc no corpo  no LOG   4/12/22"
    # "Rocket Dynamics"
    # "TVA plant predictor and\ninertial to body"
    # "HOUSEKEEPING DATA (German TVA)"
    # "TVA"
    # "Simulation"
    # "Euler Angles to table"
    # "Integration"
    # "INS"
    # "DEG"
    # "True = Civita info\nfalse = sim info"
    # "0 - Constant values\n1 - Received TVA cmds\n2 - Simulated control"
    # "Control"
    # "DMARS data"
    # "Rotation integration"
    # "Translation integration"
    # "Time"
    # "Vehicle parameters"
    n207 = node-c288() -> (w517:i64, w650:i64)  [unwired: 1 in]
    "Iteration Duration sim [us]" <- w517
    n208 = Unbundle By Name(w490) -> ("Sim_Time [s]"=w540:dbl)
    "Sim_Time [s]" <- w540
    n209 = Unbundle By Name(w490) -> ("Control Selection"=w522:enum16{"Constant", "TVA E-BOX", "Sim Control"}, "CFN-61G Enable"=w541:bool)
    n210 = case shown="True" w519 {
      tunnel: [w656 "Start_SIMULATION"] -> w521
      tunnel: [w655 "stop RT"] -> w520
      frame False {
        n211 = shared-variable "NI-PXI8106\\Library 1.lvlib\\stop SIM"() -> (w655:bool)  [unwired: 1 in, 1 out]
        n212 = shared-variable "NI-PXI8106\\Library 1.lvlib\\Run_SIM"() -> (w656:bool)  [unwired: 1 in, 1 out]
      }
      frame True {
      }
    }
    n213 = Greater?(x=w517, y=i64 5000) -> (0:→"bad iteration":bool)
    n214 = Unbundle By Name(w539) -> ("dl [º]"=w538:dbl, "Nozzle misalignment yaw/pitch [º]"=w537:dbl[], "Nozzle eccentricity x/y [m]"=w536:dbl[])
    n215 = call "Time (SubVI).vi"("Period"=w650, "Sim_Time [s]"=w540, "stop RT"=w520, "Run_SIMULATION"=w521) -> ("Stop"=w524:bool, "SIM_Running"=→"SIM_Running":bool, "i, sim_running, t[s], dt[s]"=w479:T14, "Sim t [s]"=→"Current time [s]":dbl)  [unwired: 4 in]
    n216 = Unbundle By Name(w479) -> ("t[s]"=w478:dbl)
    n217 = Unbundle By Name(w490) -> ("CFN-61G Enable"=w542:bool)
    n218 = Unbundle By Name(w479) -> ("sim_running"=w567:bool)
    n219 = shared-variable ".\\Library 1.lvlib\\XYZ - rate_CIVITA [rad_s]"() -> (w619:sgl[])  [unwired: 1 in, 1 out]
    n220 = shared-variable ".\\Library 1.lvlib\\Stop_RT"(w524) -> ()  [unwired: 1 in, 1 out]
    n221 = Unbundle By Name(w479) -> ("sim_running"=w489:bool, "t[s]"=w598:dbl)
    n222 = shared-variable ".\\Library 1.lvlib\\Euler Angles_CIVITA"() -> (w621:sgl[])  [unwired: 1 in, 1 out]
    n223 = call "Vehicle Parameters (SubVI).vi"("Nozzle eccentricity x/y [m] in"=w536, "Nozzle misalignment yaw/pitch [º] in"=w537, "dl [º]"=w538) -> ("Vehicle Parameters"=w485:T15)  [unwired: 8 in]
    n224 = Index Array(array=w619, index #1=0 ("index")) -> (element #1=w617:sgl, element #2=w615:sgl, element #3=w616:sgl)  [unwired: 2 in]
    n225 = Not(x=w567) -> (.not. x?=w566:bool)
    n226 = Negate(x=w615) -> (-x=w614:sgl)
    n227 = call "CIVITA_DMARS_conv_PXI(SubVI).vi"("Initial Euler Angles [rad]"=w528, "SIM_start"=w566, "Civitanav readings [deg]"=w621) -> ("Euler Angles [rad]"=w544:cluster{"phi":dbl, "theta":dbl, "psi":dbl})  [unwired: 5 in, 3 out]
    n228 = Build Array(w616, w614, w617) -> (w613:sgl[])
    n229 = call "Euler_ang2quat RAD(SubVI).vi"("Euler Angles [rad]"=w544) -> ("Quaternions"=w620:dbl[])  [unwired: 10 in]
    n230 = To Double Precision Float(number=w613) -> (double precision float=w612:dbl[])
    n231 = expression code="(x/pi)*180.0" "radians to degrees"(w544) -> (w518:cluster{"phi":dbl, "theta":dbl, "psi":dbl})
    "CIVITA as DMARS [º]" <- w518
    n232 = feedback #1(dbl[] [0.0, 0.0]) -> (w491:dbl[])
    n233 = shared-variable ".\\Library 1.lvlib\\TVA cmd [rad]"(w491) -> ()  [unwired: 1 in, 1 out]
    n234 = shared-variable ".\\Library 1.lvlib\\CIVITA as DMARS [º]"(w518) -> ()  [unwired: 1 in, 1 out]
    n235 = shared-variable ".\\Library 1.lvlib\\Roll Rate_angle"() -> (w551:dbl[])  [unwired: 1 in, 1 out]
    n236 = call "roll rate_angle(SubVI).vi"("Roll Rate/angle [deg]"=w551) -> ("Roll Angle[rad]"=w549:dbl[], "Roll Rate[rad/s]"=w550:dbl[])  [unwired: 9 in]
    n237 = Build Array(w550, w549) -> (w548:dbl[][])
    n238 = Not(x=w489) -> (.not. x?=w498:bool)
    n239 = Unbundle By Name(w490) -> ("German TVA Enable"=w504:bool)
    n240 = shared-variable ".\\Library 1.lvlib\\BR ACT [rad]"() -> (w506:dbl[])  [unwired: 1 in, 1 out]
    n241 = Unbundle By Name(w490) -> ("BR ACT enable"=w507:bool)
    n242 = shared-variable ".\\Library 1.lvlib\\Act_b_225_315"() -> (w502:dbl[])  [unwired: 1 in, 1 out]
    n243 = Select(t=w506, s=w507, f=w491) -> (s? t:f=w508:dbl[])
    n244 = expression code="(x/180.0)*pi" ("degrees to radians")(w502) -> (w497:dbl[])
    n245 = expression code="(x/pi)*180.0" "radians to degrees"(w528) -> (w527:cluster{"phi":dbl, "theta":dbl, "psi":dbl})
    n246 = Unbundle By Name(w490) -> ("V_ini [m/s]"=w564:dbl[], "latd_ini [º]"=w563:dbl, "lon_ini [º]"=w562:dbl, "altitude_ini(m)"=w561:dbl)
    n247 = Unbundle By Name(w490) -> ("W_b ini [rad/s]"=w560:dbl[], "W ini [rad/s]"=w559:dbl[])
    n248 = Unbundle By Name(w479) -> ("dt [s]"=w525:dbl, "sim_running"=w572:bool)
    n249 = Unbundle By Name(w479) -> ("t[s]"=w523:dbl, "sim_running"=w535:bool)
    n250 = call "Euler_ang2quat(SubVI).vi"("Euler Angles [deg]"=w527) -> ("Quaternions"=w588:dbl[])  [unwired: 10 in]
    n251 = Not(x=w572) -> (.not. x?=w573:bool)
    n252 = expression code="(x/180.0)*pi" "degrees to radians"(w563) -> (w637:dbl)
    n253 = expression code="(x/180.0)*pi" "degrees to radians"(w562) -> (w634:dbl)
    n254 = feedback #2(w560) -> (w632:dbl[])
    n255 = Select(t=w560, s=w573, f=w632) -> (s? t:f=w585:dbl[])
    n256 = feedback #3(w559) -> (w625:dbl[])
    n257 = Select(t=w559, s=w573, f=w625) -> (s? t:f=w607:dbl[])
    n258 = feedback #4(w588) -> (w631:dbl[])
    n259 = Select(t=w588, s=w573, f=w631) -> (s? t:f=w592:dbl[])
    n260 = call "RT_q2DCM (SubVI).vi"("Quaternion"=w592) -> ("DCM"=w591:dbl[][])  [unwired: 10 in]
    n261 = call "Sub_predictor_v4(SubVI).vi"("predicted step"=w623, "Sim_running"=w535, "q_i"=w592, "Pred ?"=w589, "t [s]"=w523) -> ("Euler Angles Table_pred [deg]"=w622:dbl[], "DMARS SIM pred [º]"=→"DMARS SIM pred[º]":cluster{"phi":dbl, "theta":dbl, "psi":dbl})  [unwired: 3 in, 2 out]
    "Table cmd [º] inner middle outer" <- w622
    n262 = call <vilib>:"Direction Cosines To Euler Angles.vi"("rotation order"=w644, "Direction Cosines"=w591) -> ("Euler Angles"=w641:cluster{"phi":dbl, "theta":dbl, "psi":dbl})  [unwired: 8 in, 1 out]
    n263 = shared-variable ".\\Library 1.lvlib\\Euler Angles Table [deg]"(w622) -> ()  [unwired: 1 in, 1 out]
    n264 = Unbundle(w641) -> ("phi"=w643:dbl, "theta"=w642:dbl, "psi"=w640:dbl)
    n265 = feedback #5(w564) -> (w636:dbl[])
    n266 = Select(t=w564, s=w573, f=w636) -> (s? t:f=w597:dbl[])
    n267 = feedback #6(w637) -> (w638:dbl)
    n268 = Select(t=w637, s=w573, f=w638) -> (s? t:f=w586:dbl)
    n269 = feedback #7(w634) -> (w635:dbl)
    n270 = Select(t=w634, s=w573, f=w635) -> (s? t:f=w587:dbl)
    n271 = feedback #8(w561) -> (w633:dbl)
    n272 = Select(t=w561, s=w573, f=w633) -> (s? t:f=w599:dbl)
    n273 = Build Array(w643, w642, w640) -> (w526:dbl[])
    n274 = Bundle By Name ("importante para o inicio")(cluster="Rotation", "W_b(i) [rad/s]"=w585, "W(i) [rad/s]"=w607, "q(i)"=w592, "Euler Angles {rad]"=w526) -> (w484:T3)
    n275 = Unbundle By Name(w484) -> ("q(i)"=w575:dbl[])
    n276 = Unbundle By Name(w484) -> ("W_b(i) [rad/s]"=w543:dbl[], "q(i)"=w568:dbl[])
    n277 = call "RT_q2DCM (SubVI).vi"("Quaternion"=w575) -> ("DCM"=w576:dbl[][])  [unwired: 10 in]
    n278 = call-poly <vilib>:"Array To Matrix.vi"("Real 2D Array"=w576) -> ("Real Matrix"=w577:T16)
    n279 = Select(t=w620, s=w542, f=w568) -> (s? t:f=w530:dbl[])
    n280 = Select(t=w612, s=w542, f=w543) -> (s? t:f=w545:dbl[])
    n281 = call "quat2eulerXYZ.vi"("Quaternions"=w530) -> ("Euler Angles [rad]"=w529:cluster{"phi":dbl, "theta":dbl, "psi":dbl})  [unwired: 10 in]
    n282 = Unbundle(w529) -> ("phi"=w534:dbl, "theta"=w533:dbl, "psi"=w532:dbl)
    n283 = Build Array(w534, w533, w532) -> (w531:dbl[])
    n284 = Build Array(w545, w531) -> (w546:dbl[][])
    n285 = Select(t=w548, s=w547, f=w546) -> (s? t:f=w492:dbl[][])
    n286 = Index Array(array=w492) -> (element #1=w503:dbl[], element #2=w499:dbl[])  [unwired: 4 in]
    n287 = call "Act_cmd_2 (SubVI).vi"("W_b [rad/s]"=w503, "Euler Angles [rad]"=w499, "TVA_cmd [rad]"=w508) -> ("Act315_Act225"=w510:dbl[])  [unwired: 7 in, 1 out]
    n288 = case shown="False" w507 {
      tunnel: [w653 w654] -> w509
      tunnel: w510 -> [w651 w654]
      tunnel: w498 -> [w652 _]
      frame False {
        # "TVA plant"
        n289 = call "RT_Act_Plant_5ms_2_v1 (SubVI).vi"("not.Sim_Running"=w652, "TVA_cmd"=w651) -> ("Act_b"=w653:dbl[])  [unwired: 7 in, 2 out]
      }
      frame True {
      }
    }
    n290 = Index Array(array=w499, index=2) -> (element=w495:dbl)
    n291 = call "RT_TVAr_i (SubVI).vi"("roll1"=w495, "Act315_Act225"=w497) -> ("TVA_p/TVA_y"=w496:dbl[])  [unwired: 13 in]
    n292 = expression code="(x/pi)*180.0" ("radians to degrees")(w496) -> (w494:dbl[])
    n293 = Select(t=w497, s=w504, f=w509) -> (s? t:f=w505:dbl[])
    n294 = call "Oil_Consumption (SubVI).vi"("act_b"=w505, "not.Sim_Running"=w498) -> ("Oil Consumption [L]"=w501:dbl)  [unwired: 9 in]
    n295 = Bundle By Name(cluster=T9 {"act_b [rad]"=[], "Oil Consumption [L]"=0.0, "Act_b_TVA (315,225) [deg]"=[], "TVA cmd [rad]"=[], "BR ACT [rad]"=[]} ("TVA"), "Act_b_TVA (315,225) [deg]"=w502, "Oil Consumption [L]"=w501, "act_b [rad]"=w505, "BR ACT [rad]"=w506, "TVA cmd [rad]"=w491) -> (w488:T9)
    n296 = shared-variable ".\\Library 1.lvlib\\TVA_p_TVA_y_rec"(w494) -> ()  [unwired: 1 in, 1 out]
    n297 = shared-variable ".\\Library 1.lvlib\\Act_b_rad"(w505) -> ()  [unwired: 1 in, 1 out]
    n298 = disable-structure shown="Disabled" {
      frame Disabled {
        (unwired) dbl[] [0.9999619154929337, 0.006684456018117924, 0.0056110787342547866, 3.750843750367606e-05]  # [0.766 - 0.643 - 0]
        (unwired) dbl[] [0.9996567767353742, 0.020067092257636514, 0.016838238751872656, 0.00033801050355844806]  # [2.3 - 1.93 - 0]
        # "Quats de atitudes iniciais"
      }
      frame Enabled {
      }
    }
    n299 = Bundle By Name ("importante para o inicio")(cluster=T12 {"latd(i) [rad]"=0.0, "lon(i) [rad]"=0.0, "height(i)(m)"=0.0, "V(i) [m/s] NWU"=[]} ("Position"), "V(i) [m/s] NWU"=w597, "latd(i) [rad]"=w586, "lon(i) [rad]"=w587, "height(i)(m)"=w599) -> (w483:T12)
    n300 = Unbundle By Name(w483) -> ("latd(i) [rad]"=w571:dbl, "lon(i) [rad]"=w570:dbl, "height(i)(m)"=w569:dbl, "V(i) [m/s] NWU"=w553:dbl[])
    n301 = Index Array(array=w553, index #1=0 ("index")) -> (element #1=w555:dbl, element #2=w557:dbl, element #3=w554:dbl)  [unwired: 2 in]
    n302 = Negate(x=w557) -> (-x=w556:dbl)
    n303 = Build Array(w555, w556, w554) -> (w552:dbl[])
    n304 = Build Array(w571, w570, w569) -> (w626:dbl[])
    n305 = call "Rocket Dynamics (SubVI).vi"("TVA"=w488, "Data"=w487, "V_Wind [m/s]"=w486, "Vehicle Param"=w485, "Time"=w479, "Rotation"=w484, "Position"=w483, "Fe_data"=w482) -> ("output Rocket Dynamics"=w477:T17)  [unwired: 19 in]
    n306 = Unbundle By Name(w477) -> ("acc [m/s^2]"=w511:dbl[])
    n307 = call-poly <vilib>:"Array To Matrix.vi"("Real 1D Array"=w511) -> ("Real Matrix (Column Vector)"=w578:T16)
    n308 = Unbundle By Name(w477) -> ("k_acc.lat_acc_mod"=w476:dbl, "k_acc.up_acc"=w475:dbl)
    n309 = call-poly <vilib>:"A x B.vi"("B"=w578, "A"=w577) -> ("A x B"=w580:T16)  [unwired: 1 out]
    n310 = call-poly <vilib>:"Matrix To Array.vi"("Real Matrix"=w580) -> ("Real 2D Array"=w579:dbl[][])
    n311 = Index Array "acc_b"(array=w579, index (col)=0 ("index (row)")) -> (element=w574:dbl[])  [unwired: 1 in]
    n312 = Insert Into Array(array=dbl[] [], index=0, new element #1=w545, new element #2=w574, new element #3=w530, new element #4=w552, new element #5=w626) -> (w624:dbl[])
    n313 = disable-structure shown="Enabled" {
      disable-tunnel: w624 -> [w691 w692]
      disable-tunnel: w567 -> [w660 _]
      disable-tunnel: [w659 w692] -> w611
      frame Disabled {
        w672 = dbl[] [0.0, 0.0, 0.0, 0.0, 0.0, 0.0, 0.0, 0.0, 0.0, 0.0, 0.0, 0.0, 0.0, 0.0, 0.0, 0.0] ("TVA_cmd")
        w674 = dbl[] [0.0, 0.0, 0.0, 0.0, 0.0, 0.0, 0.0, 0.0, 0.0, 0.0, 0.0, 0.0, 0.0, 0.0, 0.0, 0.0] ("TVA_cmd")
        w675 = dbl[] [0.0, 0.0, 0.0, 0.0, 0.0, 0.0, 0.0, 0.0, 0.0, 0.0, 0.0, 0.0, 0.0, 0.0, 0.0, 0.0] ("TVA_cmd")
        w676 = dbl[] [0.0, 0.0, 0.0, 0.0, 0.0, 0.0, 0.0, 0.0, 0.0, 0.0, 0.0, 0.0, 0.0, 0.0, 0.0, 0.0] ("TVA_cmd")
        w677 = dbl[] [0.0, 0.0, 0.0, 0.0, 0.0, 0.0, 0.0, 0.0, 0.0, 0.0, 0.0, 0.0, 0.0, 0.0, 0.0, 0.0] ("TVA_cmd")
        w683 = dbl[] [0.0, 0.0, 0.0, 0.0, 0.0, 0.0, 0.0, 0.0, 0.0, 0.0, 0.0, 0.0, 0.0, 0.0, 0.0, 0.0] ("TVA_cmd")
        w685 = dbl[] [0.0, 0.0, 0.0, 0.0, 0.0, 0.0, 0.0, 0.0, 0.0, 0.0, 0.0, 0.0, 0.0, 0.0, 0.0, 0.0] ("TVA_cmd")
        w687 = dbl[] [0.0, 0.0, 0.0, 0.0, 0.0, 0.0, 0.0, 0.0, 0.0, 0.0, 0.0, 0.0, 0.0, 0.0, 0.0, 0.0] ("TVA_cmd")
        w689 = dbl[] [0.0, 0.0, 0.0, 0.0, 0.0, 0.0, 0.0, 0.0, 0.0, 0.0, 0.0, 0.0, 0.0, 0.0, 0.0, 0.0] ("TVA_cmd")
        w686 = dbl[] [0.0, 0.0, 0.0, 0.0, 0.0, 0.0, 0.0, 0.0, 0.0, 0.0, 0.0, 0.0, 0.0, 0.0, 0.0, 0.0] ("TVA_b")
        # "Simulated DMARS"
        n314 = feedback #9(w689) -> (w690:dbl[])
        n315 = Select(t=w689, s=w660, f=w690) -> (s? t:f=w682:dbl[])
        n316 = feedback-in #9(w691) -> ()
        n317 = feedback #10(w687) -> (w688:dbl[])
        n318 = Select(t=w687, s=w660, f=w688) -> (s? t:f=w681:dbl[])
        n319 = feedback-in #10(w682) -> ()
        n320 = feedback #11(w685) -> (w671:dbl[])
        n321 = Select(t=w685, s=w660, f=w671) -> (s? t:f=w666:dbl[])
        n322 = feedback-in #11(w681) -> ()
        n323 = feedback #12(w677) -> (w670:dbl[])
        n324 = Select(t=w677, s=w660, f=w670) -> (s? t:f=w665:dbl[])
        n325 = feedback-in #12(w666) -> ()
        n326 = feedback #13(w676) -> (w669:dbl[])
        n327 = Select(t=w676, s=w660, f=w669) -> (s? t:f=w664:dbl[])
        n328 = feedback-in #13(w665) -> ()
        n329 = feedback #14(w675) -> (w668:dbl[])
        n330 = Select(t=w675, s=w660, f=w668) -> (s? t:f=w663:dbl[])
        n331 = feedback-in #14(w664) -> ()
        n332 = feedback #15(w674) -> (w667:dbl[])
        n333 = Select(t=w674, s=w660, f=w667) -> (s? t:f=w661:dbl[])
        n334 = feedback-in #15(w663) -> ()
        n335 = feedback #16(w672) -> (w673:dbl[])
        n336 = Select(t=w672, s=w660, f=w673) -> (s? t:f=w662:dbl[])
        n337 = feedback-in #16(w661) -> ()
        n338 = feedback #17(w683) -> (w684:dbl[])
        n339 = Select(t=w683, s=w660, f=w684) -> (s? t:f=w680:dbl[])
        n340 = feedback #18(w686) -> (w678:dbl[])
        n341 = Select(t=w686, s=w660, f=w678) -> (s? t:f=w679:dbl[])
        n342 = call "RT_DMARS (SubVI).vi"("y2"=w679, "y1"=w680, "u8"=w662, "u7"=w661) -> ("DMARS Data"=w659:dbl[])  [unwired: 7 in]
        n343 = feedback-in #17(w659) -> ()
        n344 = feedback-in #18(w680) -> ()
      }
      frame Enabled {
      }
    }
    n345 = shared-variable ".\\Library 1.lvlib\\DMARS"(w611) -> ()  [unwired: 1 in, 1 out]
    n346 = Unbundle By Name(w477) -> ("acc [m/s^2]"=w512:dbl[])
    n347 = Unbundle By Name(w477) -> ("ang_acc"=w513:dbl[])
    n348 = call "RT_Rotation_Integration_v2 (SubVI).vi"("W_b(i) [rad/s]"=w585, "ang_acc [rad/s^2]"=w513, "q(i) in"=w592, "dt"=w525) -> ("W(i+1)"=w603:dbl[], "W_b(i+1) [rad/s]"=w602:dbl[], "q(i+1)"=w601:dbl[], "Euler angles (i+1) XYZ [rad]"=w600:dbl[])  [unwired: 12 in]
    n349 = feedback-in #2(w602) -> ()
    n350 = feedback-in #3(w603) -> ()
    n351 = feedback-in #4(w601) -> ()
    n352 = call "Translation_Integration2.vi"("acc"=w512, "V(i) in"=w597, "latd(i)"=w586, "lon(i) [rad]"=w587, "height(i) [m]"=w599, "dt [s]"=w525) -> ("position"=w639:dbl[], "position ECEF (i) [m]"=w609:dbl[], "Lat_C [rad]"=w608:dbl, "Velocity"=w596:dbl[])  [unwired: 10 in]
    n353 = feedback-in #5(w596) -> ()
    n354 = Bundle By Name(cluster=T10 {"W(i+1) [rad/s]"=[], "W_b(i+1) [rad/s]"=[], "q(i+1)"=[], "Euler angles (i+1) XYZ [rad]"=[]} ("output cluster 2"), "W(i+1) [rad/s]"=w603, "W_b(i+1) [rad/s]"=w602, "q(i+1)"=w601, "Euler angles (i+1) XYZ [rad]"=w600) -> (w590:T10)
    n355 = Index Array(array=w639, index #1=0 ("index")) -> (element #1=w606:dbl, element #2=w605:dbl, element #3=w604:dbl)  [unwired: 2 in]
    n356 = feedback-in #6(w606) -> ()
    n357 = feedback-in #7(w605) -> ()
    n358 = feedback-in #8(w604) -> ()
    n359 = Bundle By Name(cluster=T11 {"position ECEF (i)"=[], "Lat_C [rad]"=0.0, "latd(i+1) [rad]"=0.0, "lon(i+1) [rad]"=0.0, "height (i+1) [m]"=0.0, "V(i+1) [m/s] NWU"=[]} ("output cluster 2"), "position ECEF (i)"=w609, "Lat_C [rad]"=w608, "latd(i+1) [rad]"=w606, "lon(i+1) [rad]"=w605, "height (i+1) [m]"=w604, "V(i+1) [m/s] NWU"=w596) -> (w514:T11)
    n360 = case shown="\"Sim Control\"" w522 {
      tunnel: [w694 w700 w734] -> w630
      tunnel: [w693 w701 w733] -> w629
      tunnel: w487 -> [_ _ w730]
      tunnel: w598 -> [_ w699 w737]
      tunnel: w584 -> [_ _ w744]
      tunnel: w544 -> [_ _ w725]
      tunnel: w489 -> [_ w702 w727]
      tunnel: w590 -> [_ _ w731]
      tunnel: w483 -> [_ _ w732]
      tunnel: w479 -> [_ _ w729]
      tunnel: w484 -> [_ _ w728]
      tunnel: w541 -> [_ _ w724]
      tunnel: w514 -> [_ _ w723]
      tunnel: w477 -> [_ _ w722]
      tunnel: w481 -> [_ _ w720]
      tunnel: [_ _ w719] -> w480
      frame "Constant", Default {
        w693 = 0.0  # Pitch
        w694 = 0.0  # Yaw
      }
      frame "TVA E-BOX" {
        w709 = T18 2 items=["1-norm"=1, "2-norm"=2, "Inf-norm"=3, "-Inf-norm"=4, "User Defined"=5] ("norm type")
        n361 = shared-variable ".\\Library 1.lvlib\\TVA"() -> (w696:dbl[])  [unwired: 1 in, 1 out]
        "TVA_cmd [deg] 2" <- w696
        n362 = call-poly <vilib>:"Vector Norm.vi"("norm type"=w709, "Input Vector"=w696) -> ("norm"=w695:dbl)  [unwired: 8 in, 1 out]
        n363 = Divide(x=w696, y=w695) -> (x/y=w704:dbl[])
        n364 = Greater?(x=w695, y=3.0) -> (0:w706:bool)
        n365 = Multiply(x=3.0 ("y"), y=w704) -> (x*y=w703:dbl[])
        n366 = Select(t=w703, s=w706, f=w696) -> (s? t:f=w707:dbl[])
        n367 = Index Array(array=w707, index #1=0 ("index")) -> (element #1=w698:dbl, element #2=w697:dbl)  [unwired: 1 in]
        n368 = disable-structure shown="Enabled" {
          disable-tunnel: w702 -> [w716 _]
          disable-tunnel: [w715 w718] -> w701
          disable-tunnel: [w714 w717] -> w700
          disable-tunnel: w699 -> [w713 _]
          disable-tunnel: w698 -> [w712 w718]
          disable-tunnel: w697 -> [w711 w717]
          frame Disabled {
            n369 = call "TVA_cmd_LMS(SubVI).vi"("t [s]"=w713, "Sim_running"=w716, "TVA_yaw"=w711, "TVA_pitch"=w712) -> ("TVA_yaw_LMS"=w714:dbl, "TVA_pitch_LMS"=w715:dbl)  [unwired: 6 in]
          }
          frame Enabled {
          }
        }
      }
      frame "Sim Control" {
        # "Tentativa de eliminar porradas (Euler)"
        n370 = Quotient & Remainder(x=w744, y=2) -> (x-y*floor(x/y)=w742:i32)  [unwired: 1 out]
        n371 = Not Equal To 0?(x=w742) -> (x != 0?=w740:bool)
        n372 = call "Control_3.vi"("latd-lon-heig-VNWU"=w732, "CIVITA as DMARS [rad]"=w725, "Guiamento"="Guiamento", "PID_array"=w720, "Wi1-Wbi1-qi1-Euli1"=w731, "Civita?"=w724, "output Rocket Dynamics"=w722, "File"=w730, "dt-sim_run-t-i"=w729, "Position (i+1)"=w723, "Rotation"=w728, "sim_running"=w727) -> ("TVA_cmd(i+1,:) [deg]"=w726:dbl[], "e(i+1)"=w719:dbl[])  [unwired: 1 in, 1 out]
        n373 = Index Array(array=w726, index #1=0 ("index")) -> (element #1=w741:dbl, element #2=w738:dbl)  [unwired: 1 in]
        n374 = case shown="False" FALSE {
          tunnel: [w756 w781] -> w736
          tunnel: [w755 w780] -> w735
          tunnel: w741 -> [w757 w779]
          tunnel: w738 -> [w754 w778]
          tunnel: w740 -> [_ w777]
          frame False {
            n375 = disable-structure shown="Enabled" {
              disable-tunnel: w757 -> [w767 w775]
              disable-tunnel: [w766 w775] -> w756
              disable-tunnel: [w760 w774] -> w755
              disable-tunnel: w754 -> [w759 w774]
              frame Disabled {
                n376 = feedback #19(w759) -> (w758:dbl)
                n377 = feedback-in #19(w759) -> ()
                n378 = feedback #20(w767) -> (w768:dbl)
                n379 = feedback-in #20(w767) -> ()
                n380 = Absolute Value(x=w758) -> (abs(x)=w763:dbl)
                n381 = Absolute Value(x=w768) -> (abs(x)=w771:dbl)
                n382 = Absolute Value(x=w759) -> (abs(x)=w762:dbl)
                n383 = Absolute Value(x=w767) -> (abs(x)=w772:dbl)
                n384 = Multiply(x=5.0, y=w763) -> (x*y=w765:dbl)
                n385 = Multiply(x=5.0, y=w771) -> (x*y=w769:dbl)
                n386 = Greater Or Equal?(x=w772, y=w769) -> (x >= y?=w773:bool)
                n387 = Greater Or Equal?(x=w762, y=w765) -> (x >= y?=w761:bool)
                n388 = Select(t=w768, s=w773, f=w767) -> (s? t:f=w766:dbl)
                n389 = Select(t=w758, s=w761, f=w759) -> (s? t:f=w760:dbl)
              }
              frame Enabled {
              }
            }
          }
          frame True {
            # "10ms output"
            n390 = feedback #21(w779) -> (w776:dbl)
            n391 = feedback #22(w778) -> (w782:dbl)
            n392 = Select(t=w779, s=w777, f=w776) -> (s? t:f=w781:dbl)
            n393 = feedback-in #21(w781) -> ()
            n394 = Select(t=w778, s=w777, f=w782) -> (s? t:f=w780:dbl)
            n395 = feedback-in #22(w780) -> ()
          }
        }
        n396 = disable-structure shown="Enabled" {
          disable-tunnel: w727 -> [w751 _]
          disable-tunnel: w737 -> [w750 _]
          disable-tunnel: w736 -> [w749 w753]
          disable-tunnel: w735 -> [w748 w752]
          disable-tunnel: [w747 w753] -> w734
          disable-tunnel: [w746 w752] -> w733
          frame Disabled {
            n397 = call "TVA_cmd_LMS(SubVI).vi"("t [s]"=w750, "Sim_running"=w751, "TVA_yaw"=w748, "TVA_pitch"=w749) -> ("TVA_yaw_LMS"=w746:dbl, "TVA_pitch_LMS"=w747:dbl)  [unwired: 6 in]
          }
          frame Enabled {
          }
        }
      }
    }
    n398 = expression code="(x/180.0)*pi" "degrees to radians"(w629) -> (w627:dbl)
    n399 = expression code="(x/180.0)*pi" "degrees to radians"(w630) -> (w628:dbl)
    n400 = Build Array(w628, w627) -> (w516:dbl[])
    n401 = feedback-in #1(w516) -> ()
    n402 = call "LOG_sim_2 (SubVI).vi"("Data File"=w487, "Rotation"=w484, "Time"=w479, "TVA"=w488, "Position"=w483, "output Rocket Dynamics"=w477) -> ()  [unwired: 6 in]
    n403 = node-c288() -> ()  [unwired: 1 in, 1 out]
  }
  n404 = Index Array(array=w14, index (col) #1=0 ("disabled index (col)")) -> (element #1=w13:dbl[], element #2=w12:dbl[], element #3=w11:dbl[])  [unwired: 5 in]
  n405 = case shown="True" "STIM300 Enable" {
    frame False {
    }
    frame True {
      w791 = FALSE  # Enable Termination Char (T)
      w792 = u32 921600  # baud rate (921600)
      # "1k sample"
      n406 = call-poly "VISA Configure Serial Port"("VISA resource name"=refnum<visa-resource-name> "COM5", "Enable Termination\nChar (T)"=w791, "baud rate (9600)"=w792) -> ("VISA resource name out"=w787:refnum<visa-resource-name>, "error out"=w788:errorcluster)  [unwired: 11 in]
      n407 = node-c288() -> (w790:T6)  [unwired: 4 in]
      n408 = timed-loop {
        timing: w790 -> [_]
        timing-out: [_] -> w789
        tunnel: w788 -> [w802]
        tunnel: w787 -> [w803]
        stop <- w794 stop-if-true
        n409 = node-c288() -> (→"Iteration Duration STIM":i64)  [unwired: 1 in]
        n410 = shared-variable ".\\Library 1.lvlib\\Stop_RT"() -> (w796:bool)  [unwired: 1 in, 1 out]
        n411 = Or(x=FALSE, y=w796) -> (x .or. y?=w794:bool)
        n412 = while {
          tunnel: w803 -> [w812]
          tunnel: w802 -> [w811]
          tunnel: [w810] -> w801
          tunnel: [w809] -> w800
          tunnel: w794 -> [w808]
          tunnel: [w804] -> w799
          tunnel: [w805] -> w798
          stop <- w806 stop-if-true
          w813 = u32 1  # byte to read
          n413 = VISA Read(VISA resource name=w812, byte count=w813, error in (no error)=w811) -> (VISA resource name out=w810:refnum<visa-resource-name>, read buffer=w804:string, error out=w809:errorcluster)  [unwired: 1 out]
          n414 = Equal?(x=w804, y="“") -> (x = y?=w805:bool)
          n415 = Or(x=w805, y=w808) -> (x .or. y?=w806:bool)
        }
        n416 = case shown="True" w798 {
          tunnel: w800 -> [_ w816]
          tunnel: w801 -> [_ w815]
          tunnel: w799 -> [_ w814]
          frame False {
          }
          frame True {
            n417 = case shown="No Error" w816 {
              selector: w816 -> [w928 _]
              tunnel: w815 -> [w927 _]
              tunnel: w814 -> [w925 _]
              frame No Error {
                w926 = u32 37  # bytes to read
                # "CRC valido para configuração x93"
                n418 = VISA Read(VISA resource name=w927, byte count=w926, error in (no error)=w928) -> (read buffer=w924:string)  [unwired: 3 out]
                n419 = Concatenate Strings(w925, w924) -> (w923:string)
                n420 = String To Byte Array(string=w923) -> (unsigned byte array=w861:u8[])
                n421 = for {
                  N: 38 -> [_]
                  tunnel: w861 -> [w929] mode=indexing
                  shift-right: [w933] -> _
                  shift-left: u32 4294967295 ("x") -> [w938]
                  shift-right: [w932] -> w913
                  shift-left: _ -> [w931]
                  i -> [w930]
                  n422 = Greater Or Equal?(x=w930, y=34) -> (x >= y?=w945:bool)
                  n423 = Select(t=u8 0, s=w945, f=w929) -> (s? t:f=w942:u8)
                  n424 = To Unsigned Long Integer(number=w942) -> (unsigned 32bit integer=w940:u32)
                  n425 = Logical Shift(y=i8 24, x=w940) -> (x << y=w939:u32)
                  n426 = Exclusive Or(1:w938, 2:w939) -> (0:w936:u32)
                  n427 = for {
                    N: 8 -> [_]
                    shift-right: [w949] -> w933
                    shift-left: w936 -> [w948]
                    n428 = Greater?(x=w948, y=u32 2147483647) -> (0:w946:bool)
                    n429 = case shown="True" w946 {
                      tunnel: w948 -> [w951 w956]
                      tunnel: [w950 w953] -> w949
                      frame False {
                        n430 = Logical Shift(y=i8 1, x=w951) -> (x << y=w950:u32)
                      }
                      frame True {
                        n431 = Logical Shift(y=i8 1, x=w956) -> (x << y=w955:u32)
                        n432 = Exclusive Or(1:u32 79764919, 2:w955) -> (0:w953:u32)
                      }
                    }
                  }
                  n433 = Equal?(x=w930, y=35) -> (x = y?=w935:bool)
                  n434 = Select(t=w933, s=w935, f=w931) -> (s? t:f=w932:u32)
                }
                n435 = Index Array(array=w861, index #1=34 ("index")) -> (element #1=w919:u8, element #2=w920:u8, element #3=w921:u8, element #4=w922:u8)  [unwired: 3 in]
                n436 = Join Numbers(hi=w921, lo=w922) -> ((hi.lo)=w916:u16)
                n437 = Join Numbers(hi=w919, lo=w920) -> ((hi.lo)=w917:u16)
                n438 = Join Numbers(hi=w917, lo=w916) -> ((hi.lo)=w912:u32)
                n439 = Equal?(x=w912, y=w913) -> (x = y?=w859:bool)
                "CRC OK" <- w859
                n440 = Index Array(array=w861, index #1=1 ("index")) -> (element #1=w907:u8, element #2=w899:u8, element #3=w900:u8, element #4=w901:u8, element #5=w902:u8, element #6=w903:u8, element #7=w904:u8, element #8=w905:u8, element #9=w906:u8, element #10=w832:u8)  [unwired: 9 in]
                "IMU gyro status" <- w832
                n441 = Index Array(array=w861, index #1=21 ("index")) -> (element #1=w875:u8, element #2=w867:u8, element #3=w868:u8, element #4=w869:u8, element #5=w870:u8, element #6=w871:u8, element #7=w872:u8, element #8=w873:u8, element #9=w874:u8, element #10=w877:u8)  [unwired: 9 in]
                "IMU incl status" <- w877
                n442 = Index Array(array=w861, index=31) -> (element=w834:u8)
                "Samples Counter" <- w834
                n443 = Index Array(array=w861, index #1=11 ("index")) -> (element #1=w882:u8, element #2=w890:u8, element #3=w889:u8, element #4=w888:u8, element #5=w887:u8, element #6=w886:u8, element #7=w885:u8, element #8=w884:u8, element #9=w883:u8, element #10=w880:u8)  [unwired: 9 in]
                "IMU accel status" <- w880
                n444 = Equal?(x=w832, y=u8 0) -> (x = y?=w908:bool)
                n445 = Equal?(x=w877, y=u8 0) -> (x = y?=w876:bool)
                n446 = Equal?(x=w880, y=u8 0) -> (x = y?=w881:bool)
                n447 = Build Array(w907, w899, w900) -> (w898:u8[])
                n448 = Build Array(w901, w902, w903) -> (w896:u8[])
                n449 = Build Array(w904, w905, w906) -> (w897:u8[])
                n450 = And(x=w908, y=w859) -> (x .and. y?=w895:bool)
                n451 = Build Array(w875, w867, w868) -> (w866:u8[])
                n452 = Build Array(w869, w870, w871) -> (w864:u8[])
                n453 = Build Array(w872, w873, w874) -> (w865:u8[])
                n454 = Build Array(w882, w890, w889) -> (w891:u8[])
                n455 = Build Array(w888, w887, w886) -> (w893:u8[])
                n456 = Build Array(w885, w884, w883) -> (w892:u8[])
                n457 = And(x=w876, y=w859) -> (x .and. y?=w863:bool)
                n458 = And(x=w881, y=w859) -> (x .and. y?=w894:bool)
                n459 = To Double Precision Float(number=w834) -> (double precision float=w833:dbl)
                n460 = call "ConversaoP (SubVI).vi"("Valido?"=w895, "Z"=w897, "Y"=w896, "X"=w898) -> ("Z"=w853:dbl, "Y"=w854:dbl, "X"=w855:dbl)  [unwired: 5 in]
                n461 = call "ConversaoP (SubVI).vi"("Valido?"=w863, "Z"=w865, "Y"=w864, "X"=w866) -> ("Z"=w847:dbl, "Y"=w846:dbl, "X"=w848:dbl)  [unwired: 5 in]
                n462 = call "ConversaoP (SubVI).vi"("Valido?"=w894, "Z"=w892, "Y"=w893, "X"=w891) -> ("Z"=w844:dbl, "Y"=w843:dbl, "X"=w845:dbl)  [unwired: 5 in]
                n463 = Scale By Power Of 2(n=i8 14, x=1.0) -> (x*2^n=w857:dbl)
                n464 = Scale By Power Of 2(n=i8 19, x=1.0) -> (x*2^n=w852:dbl)
                n465 = Scale By Power Of 2(n=i8 22, x=1.0) -> (x*2^n=w849:dbl)
                n466 = Divide(x=w855, y=w857) -> (x/y=w840:dbl)
                n467 = Divide(x=w854, y=w857) -> (x/y=w839:dbl)
                n468 = Divide(x=w853, y=w857) -> (x/y=w838:dbl)
                n469 = Divide(x=w845, y=w852) -> (x/y=w837:dbl)
                n470 = Divide(x=w843, y=w852) -> (x/y=w836:dbl)
                n471 = Divide(x=w844, y=w852) -> (x/y=w835:dbl)
                n472 = Divide(x=w848, y=w849) -> (x/y=w830:dbl)
                "Inc X [g]" <- w830
                n473 = Divide(x=w846, y=w849) -> (x/y=w828:dbl)
                "Inc Y [g]" <- w828
                n474 = Divide(x=w847, y=w849) -> (x/y=w827:dbl)
                "Inc Z [g]" <- w827
                n475 = Inverse Tangent (2 Input)(1:w827, 2:w828) -> (0:w829:dbl)
                n476 = Inverse Tangent (2 Input)(1:w827, 2:w830) -> (0:w831:dbl)
                n477 = Build Array(w840, w839, w838, w837, w836, w835, w830, w828, w827, w833) -> ()  [unwired: 1 out]
                n478 = expression code="(x/pi)*180.0" "radians to degrees"(w829) -> (w823:dbl)
                n479 = expression code="(x/pi)*180.0" "radians to degrees"(w831) -> (w824:dbl)
                n480 = Negate(x=-0.5664464386142395 ("mean y")) -> (-x=w825:dbl)
                n481 = Negate(x=-0.5804380367688414 ("mean x")) -> (-x=w826:dbl)
                n482 = Add(x=w825, y=w823) -> (x+y=w817:dbl)
                "Incl angle Y [deg]" <- w817
                n483 = Add(x=w826, y=w824) -> (x+y=w820:dbl)
                "Incl angle X [deg]" <- w820
                n484 = call <vilib>:"Mean PtByPt.vi"("x"=w817) -> ("mean"=→"mean y":dbl)  [unwired: 3 in, 1 out]
                n485 = call <vilib>:"Mean PtByPt.vi"("x"=w820) -> ("mean"=→"mean x":dbl)  [unwired: 3 in, 1 out]
              }
              frame Error {
              }
            }
          }
        }
        n486 = node-c288() -> ()  [unwired: 1 in, 1 out]
      }
      n487 = node-c288(w789) -> ()  [unwired: 1 out]
    }
  }
  n488 = Bundle(w1, "e(i+1)"=w12) -> (w8:cluster{dbl[], "e(i+1)":dbl[]})  [unwired: 1 in]
  n489 = Bundle(w1, "e(i+1)"=w13) -> (w10:cluster{dbl[], "e(i+1)":dbl[]})  [unwired: 1 in]
  n490 = Bundle(w1, "e(i+1)"=w11) -> (w9:cluster{dbl[], "e(i+1)":dbl[]})  [unwired: 1 in]
  n491 = Bundle(w1, w5) -> (w3:cluster{dbl[], dbl[]})  [unwired: 1 in]
  n492 = Bundle(w1, w4) -> (w2:cluster{dbl[], dbl[]})  [unwired: 1 in]
  n493 = Build Array(w10, w8, w9, w3, w2) -> (→"e (i+1)":cluster{dbl[], "e(i+1)":dbl[]}[])
  n494 = Unbundle By Name(w27) -> ("LOG Enable"=w29:bool)
  "LOG Enable" <- w29
  n495 = case shown="True" w29 {
    frame False {
    }
    frame True {
      # "LOG"
      n496 = flat-sequence {
        tunnel: [w968] -> w966
        tunnel: [w967] -> w964
        tunnel: w966 -> [w995]
        tunnel: [w995] -> w965
        tunnel: w964 -> [w994]
        tunnel: [w994] -> w963
        tunnel: w965 -> [w1003]
        tunnel: w963 -> [w1002]
        frame #0 {
          n497 = disable-structure shown="Enabled" {
            disable-tunnel: [w980 w991] -> w968
            disable-tunnel: [w978 w989] -> w967
            frame Disabled {
              # "Path shown is for NI Linux RTOS\ntargets. VxWorks path is c:\\test1.txt"
              n498 = Get Date/Time In Seconds() -> (seconds since 1Jan1904=w971:timestamp)
              n499 = case shown="False" FALSE {
                tunnel: [".txt" ("string") ".csv" ("string")] -> w975
                frame False {
                }
                frame True {
                }
              }
              n500 = Format Date/Time String(time format string (%c)="%d%m%Y_%H%M%S", seconds (now)=w971, UTC format="UTC format") -> (date/time string=w970:string)
              n501 = Concatenate Strings(w970, w975) -> (w976:string)
              "concatenated string" <- w976
              n502 = Build Path(base path=path "c:/" ("file path (use dialog)"), name or relative path=w976) -> (appended path=w974:path)
              "appended path" <- w974
              n503 = Open/Create/Replace File(file path (use dialog)=w974, operation (0:open)=T19."replace or create") -> (refnum out=w978:refnum<file>, error out=w980:errorcluster)  [unwired: 4 in, 1 out]
            }
            frame Enabled {
              # "Path shown is for NI Linux RTOS\ntargets. VxWorks path is c:\\test1.txt"
              n504 = case shown="False" FALSE {
                tunnel: [".txt" ("string") ".csv" ("string")] -> w986
                frame False {
                }
                frame True {
                }
              }
              n505 = Concatenate Strings("LOG" ("time format string (%c)"), w986) -> (w987:string)
              "concatenated string 2" <- w987
              n506 = Build Path(base path=path "c:/" ("file path (use dialog)"), name or relative path=w987) -> (appended path=w985:path)
              "PXI log path 2" <- w985
              n507 = Open/Create/Replace File(file path (use dialog)=w985, operation (0:open)=T19."replace or create") -> (refnum out=w989:refnum<file>, error out=w991:errorcluster)  [unwired: 4 in, 1 out]
            }
          }
        }
        frame #1 {
          n508 = while {
            stop <- w996 stop-if-true
            n509 = shared-variable ".\\Library 1.lvlib\\SIM_Running"() -> (w997:bool)  [unwired: 1 in, 1 out]
            n510 = shared-variable ".\\Library 1.lvlib\\Stop_RT"() -> (w998:bool)  [unwired: 1 in, 1 out]
            n511 = Or(x=w997, y=w998) -> (x .or. y?=w996:bool)
          }
        }
        frame #2 {
          w999 = i64 5000  # Period [us]
          n512 = node-c288(w999) -> (w1005:T6)  [unwired: 3 in]
          n513 = timed-loop {
            tunnel: w1002 -> [w1017]
            tunnel: [w1016] -> w1001
            timing: w1005 -> [_]
            timing-out: [_] -> w1004
            shift-right: [w1011] -> w1000
            shift-left: w1003 -> [w1012]
            stop <- w1015 stop-if-true
            n514 = node-c288() -> (→"Iteration Duration LOG":i64)  [unwired: 1 in]
            n515 = shared-variable ".\\Library 1.lvlib\\Sim_logdata"() -> (w1010:dbl[])  [unwired: 1 in, 1 out]
            n516 = shared-variable ".\\Library 1.lvlib\\Table_LOG"() -> (w1009:dbl[])  [unwired: 1 in, 1 out]
            n517 = Insert Into Array(array=w1010, index=43, new element=w1009) -> (w1007:dbl[])
            n518 = shared-variable "NI-PXI8106\\Library 1.lvlib\\Full_LOG"(w1007) -> ()  [unwired: 1 in, 1 out]
            n519 = shared-variable ".\\Library 1.lvlib\\Stop_RT"() -> (w1015:bool)  [unwired: 1 in, 1 out]
            n520 = Array To Spreadsheet String(array=w1007, 3:"%g;" ("format string")) -> (spreadsheet string=w1013:string)  [unwired: 1 in]
            "spreadsheet string" <- w1013
            n521 = node-c288() -> ()  [unwired: 1 in, 1 out]
            n522 = Write to Text File(file (use dialog)=w1017, text=w1013, error in=w1012) -> (refnum out=w1016:refnum<file>, error out=w1011:errorcluster)  [unwired: 1 in, 1 out]
          }
          n523 = node-c288(w1004) -> ()  [unwired: 1 out]
          n524 = Close File(refnum=w1001, error in=w1000) -> ()  [unwired: 2 out]
        }
      }
    }
  }
  n525 = Unbundle By Name(w27) -> ("Table enable"=w32:bool)
  "Table enable" <- w32
  n526 = case shown="True" w32 {
    tunnel: w52 -> [_ _]
    frame False {
    }
    frame True {
      w1030 = 10000 ("timeout ms (60000)")
      w1041 = i64 5000  # Period [us]
      # "Motion Simulation Table control"
      n527 = shared-variable ".\\Library 1.lvlib\\Initial Euler Angles [deg]"() -> (w1036:cluster{"phi":dbl, "theta":dbl, "psi":dbl})  [unwired: 1 in, 1 out]
      n528 = UDP Open(9:w1030, 11:u16 9838 ("port")) -> (port=w1039:refnum<k16>, 0:w1029:errorcluster)  [unwired: 1 in, 3 out]
      n529 = TCP Open Connection(address="Remote Host", remote port or service name=u16 9878, timeout ms (60000)=w1030) -> (connection ID=w1038:refnum<k5>, error out=w1031:errorcluster)  [unwired: 2 in]
      n530 = String To IP(1:"Remote Host") -> (0:w1040:u32)
      n531 = Merge Errors(w1031, w1029) -> (w1034:errorcluster)
      n532 = call "Time Delay"("error in (no error)"=w1034) -> ("error out"=w1037:errorcluster)  [unwired: 10 in]
      n533 = node-c288(w1041) -> (w1049:T6)  [unwired: 3 in]
      n534 = call "Start_track.vi"("TCP connection ID"=w1038, "UDP connection ID"=w1039, "IP address in"=w1040, "Euler Angles DMARS [º] debug"=w1036, "error in"=w1037) -> ("TCP connection ID out"=w1042:refnum<k5>, "UDP connection ID out"=w1046:refnum<k16>, "IP address out"=w1045:u32, "error out"=w1044:errorcluster)  [unwired: 6 in, 1 out]
      n535 = timed-loop {
        timing: w1049 -> [_]
        timing-out: [_] -> w1048
        tunnel: w1046 -> [w1078]
        tunnel: w1045 -> [w1077]
        tunnel: w1044 -> [w1076]
        tunnel: [w1080] -> w1043
        tunnel: [w1079] -> w1047
        stop <- w1074 stop-if-true
        w1072 = 0
        # "Time"
        # "Send and receive table data"
        # "True when simulation starts"
        # "from predictor"
        # "Data for log file"
        n536 = node-c288() -> (w1068:i64, →"Iteration Duration TBL":i64)  [unwired: 1 in]
        "Period" <- w1068
        n537 = shared-variable ".\\Library 1.lvlib\\Euler Angles Table [deg]"() -> (w1064:dbl[])  [unwired: 1 in, 1 out]
        n538 = shared-variable ".\\Library 1.lvlib\\SIM_Running"() -> (w1065:bool)  [unwired: 1 in, 1 out]
        n539 = To Double Precision Float(number=w1068) -> (double precision float=w1069:dbl)
        n540 = Divide(x=w1069, y=1000000.0) -> (x/y=w1067:dbl)
        n541 = feedback #23(w1072) -> (w1073:i32)
        n542 = Select(t=w1073, s=w1065, f=w1072) -> (s? t:f=w1056:i32)
        n543 = call "ptbypt derivatives (SubVI).vi"("Array of Double"=w1064) -> ("outer cmd [deg]"=w1052:T20, "middle cmd [deg]"=w1062:T21, "inner cmd [deg]"=w1063:T20)  [unwired: 8 in]
        n544 = To Double Precision Float(number=w1056) -> (double precision float=w1066:dbl)
        n545 = Increment(x=w1056) -> (x+1=w1071:i32)
        n546 = feedback-in #23(w1071) -> ()
        n547 = call "Send_Demand_controlword.vi"("UDP connection ID out"=w1078, "Inner TRACK"=w1063, "Middle TRACK"=w1062, "Outer TRACK"=w1052, "IP address in"=w1077, "error in"=w1076, "ReadOnly"=FALSE) -> ("UDP connection ID out"=w1058:refnum<k16>, "concatenated string"=→"string enviada para acutrol":string, "error out"=w1060:errorcluster)  [unwired: 5 in, 1 out]
        n548 = Multiply "t [s]"(x=w1067, y=w1066) -> (x*y=w1055:dbl)
        "Time (s)" <- w1055
        n549 = shared-variable ".\\Library 1.lvlib\\Stop_RT"() -> (w1074:bool)  [unwired: 1 in, 1 out]
        n550 = call "Receive_Monitor.vi"("UDP connection ID"=w1058, "error out 2"=w1060) -> ("UDP connection ID out"=w1079:refnum<k16>, "MonitorBlock"=w1075:dbl[], "error out"=w1080:errorcluster)  [unwired: 11 in]
        n551 = Equal To 0?(x=w1055) -> (x = 0?=→"Table Ready":bool)
        n552 = call "LOG tbl (SubVI).vi"("t [s]"=w1055, "outer cmd [deg]"=w1052, "middle cmd [deg]"=w1062, "inner cmd [deg]"=w1063, "MonitorBlock"=w1075) -> ("ACCEL"=→"ACCEL":cluster{dbl, dbl, dbl}, "RATE"=→"RATE":cluster{dbl, dbl, dbl}, "POS"=→"POS":cluster{dbl, dbl, dbl})  [unwired: 4 in]
        n553 = node-c288() -> ()  [unwired: 1 in, 1 out]
      }
      n554 = node-c288(w1048) -> ()  [unwired: 1 out]
      n555 = call "Stop_Synthesis.vi"("TCP connection ID"=w1042, "error in"=w1043) -> ("TCP connection ID out"=w1027:refnum<k5>, "error out"=w1026:errorcluster)  [unwired: 12 in]
      n556 = TCP Close Connection(connection ID=w1027, error in (no error)=w1026) -> (error out=w1025:errorcluster)  [unwired: 1 in, 1 out]
      n557 = UDP Close(connection ID=w1047, 8:w1025) -> (error out=w1028:errorcluster)  [unwired: 1 out]
      n558 = call <vilib>:"General Error Handler.vi"("error in (no error)"=w1028) -> ()  [unwired: 2 in, 13 out]
    }
  }
  n559 = node-c288(w75) -> ()  [unwired: 1 out]
